vi "FLL Tournament Control.vi"() -> ()   [LabVIEW 2013]
uses:
  Team Data Array.ctl
  Team Data.ctl
  ScoreList.ctl
  Full Score Entry.ctl
  ScoreEntry.ctl
  Sound Info.ctl
  <vilib>/sound2/lvsound2.llb/Sound Data Format.ctl
  ImageInfoList.ctl
  TeamManager/TeamData_and_Schedule.ctl
  <vilib>/Utility/sysdir.llb/System Directory Type.ctl
  Logfile Entry.ctl
  Error File Queue Contents.ctl
  Score File Queue Contents.ctl
  <vilib>/sound2/lvsound2.llb/Sampling Mode.ctl
  Schedule Data.ctl
  <vilib>/Analysis/baseanly.llb/Mean (DBL).vi
  <vilib>/Utility/xml.llb/Write to XML File(string).vi
  Score Event Refnum.vi
  <vilib>/sound2/lvsound2.llb/Sound Output Set Volume (Single).vi
  <vilib>/sound2/lvsound2.llb/Sound Output Write (DBL).vi
  <vilib>/Platform/browser.llb/Open URL in Default Browser (string).vi
  <vilib>/Utility/xml.llb/Read From XML File(string).vi
  <vilib>/httpClient/LabVIEWHTTPClient.lvlib
  <vilib>/Analysis/NI_AALBase.lvlib
panel:
  in  "Local Entry Button":bool
  in  "Low Sponsor Image List":T1
  in  "Mid Sponsor Image List":T1
  in  "Top Sponsor Image List":T1
  in  "Profile Button":bool
  in  "Home Button":bool
  in  "System Monitor Button":bool
  in  "View Rankings Button":bool
  in  "Go to Timekeeper Button":bool
  in  "Launch Score Entry":bool
  in  "Settings Button":bool
  in  "Sound To Play":T2(ring)
  out "Sound Cluster":T3={"Start"={"total number of samples/ch"=31680, "sound format"={"sample rate (S/s)"=11025.0, "number of channels"=1, "bits per sample"=16}, "data"=[{"t0"=timestamp(0 s since 1904-01-01), "dt"=9.070294784580499e-05, "Y"=array[31680 elements]}], "Volume"=100.0}, "Stop"={"total number of samples/ch"=27648, "sound format"={"sample rate (S/s)"=11025.0, "number of channels"=1, "bits per sample"=16}, "data"=[{"t0"=timestamp(0 s since 1904-01-01), "dt"=9.070294784580499e-05, "Y"=array[27648 elements]}], "Volume"=100.0}, "Uh-Oh"={"total number of samples/ch"=29952, "sound format"={"sample rate (S/s)"=11025.0, "number of channels"=1, "bits per sample"=16}, "data"=[{"t0"=timestamp(0 s since 1904-01-01), "dt"=9.070294784580499e-05, "Y"=array[29952 elements]}], "Volume"=88.46153846153847}, "PreMatch"={"total number of samples/ch"=225792, "sound format"={"sample rate (S/s)"=44100.0, "number of channels"=2, "bits per sample"=16}, "data"=[{"t0"=timestamp(0 s since 1904-01-01), "dt"=2.2675736961451248e-05, "Y"=array[225792 elements]}, {"t0"=timestamp(0 s since 1904-01-01), "dt"=2.2675736961451248e-05, "Y"=array[225792 elements]}], "Volume"=75.38461538461539}, "Hurry-Up"={"total number of samples/ch"=0, "sound format"={"sample rate (S/s)"=0.0, "number of channels"=0, "bits per sample"=0}, "data"=[], "Volume"=0.0}}
  out "Table Names":string[](array[string])
  in  "Tab Control":T5(tab)=enum."Splash"
  out "Users String":string
  out "String 3":string="System Settings\n\nThis page is for Server System Settings.  \n\nTimer / Sounds - Press the button for \"Configure Sounds and Timer\" to set specific timer and sound properties.\n\nFile Paths - Don't change these unless you really know what you're doing.  If you change these, files will be saved or read from different locations than the \"default\" locations.  This may be good or bad, depending on the situation.  Beware.\n\nSecurity Entry Access Password - if you wish to put a password on the \"Web Entry\" score webpage, put the password here.  This value does not persist between software reboots.  The default value is \"321LEGO\".  When a user enters this password within the prompt when attempting to access a security-protected page, the user's \"system credentials\" are added to a Security Access List and attempts to access the software from that \"system\" no longer requires a password.  To clear out the access list and remove all users (for instance once you've set a new password to be used), press \"Clear Access List.\"  The local user ALWAYS has access."
  in  "Clear Access List Button":bool
  in  "Score Entry Access Password":string="321LEGO"
  in  "Team Data File Path":path=path "Z:/Code/LabVIEW/FLL 2.1/scorefile.xml"
  in  "Score Folder":path=path "Z:/Code/LabVIEW/FLL 2.1/Score Files"
  in  "Scoring Data File Path":path=path "Z:/Code/LabVIEW/FLL 2.1/scorefile.xml"
  in  "Timing Logfile Path":path=path "Z:/Code/LabVIEW/FLL 2.1/timing.log"
  in  "Error Folder":path=path "Z:/Code/LabVIEW/FLL 2.1/Error Files"
  in  "Error Logfile Path":path=path "Z:/Code/LabVIEW/FLL 2.1/error.log"
  in  "Scoring Logfile Path":path=path "Z:/Code/LabVIEW/FLL 2.1/scoring.log"
  in  "Schedule File Path":path=path "Z:/Code/LabVIEW/FLL 2.1/schedule.csv"
  in  "stop":bool
  in  "Configure Sounds Button":bool
  out "Timer Log":string[][](table)
  out "Scoring Log":string[][](table)
  out "Error Log":string[][](table)
  in  "PH 2":bool
  out "Score Queue Full":bool
  out "Error Queue Full":bool
  out "Write Scores to file indicator":bool
  out "Scores Exist":bool
  out "Teams Exist":bool
  out "Uh-Oh Sound Indicator":bool
  out "Stop Sound Indicator":bool
  out "Start Sound Indicator":bool
  out "Server Running":bool
  out "Web Pages Not Found":bool
  out "Log Queue Full":bool
  out "Network Interface Up":bool=TRUE
  out "PH":bool
  out "Port":string
  out "Current IP":string="192.168.0.3"
  in  "Delete Team":bool
  in  "Team Info":T6
  out "Number of Teams":i32
  in  "Score Entry":bool
  in  "Restore Session":bool
  in  "Input File Type":T8(radio)
  out "Number of Scores":i32
  in  "Replace Current Score Data\nFrom File":bool
  in  "Score File Path (Read)":path
  out "Score Data":T9 {"Score"."Score Mode Selector" items=["Automatic", "Manual"]}
  in  "Schedule To Show":enum16{"Practice", "Ranking"}(ring)=enum."Ranking"
  out "Schedule":i32(listbox)
  in  "Hurry-Up Sound Volume":dbl(slide)=88.46153846153847 scale=0.0..100.0
  in  "Hurry-Up Sound":path=path "Z:/Code/LabVIEW/FLL 2.1/sounds/FOGHORN.wav"
  out "mean":dbl format="%0.2f"
  out "min value":u32
  out "max value":u32
  in  "Boolean":bool
  in  "Secondary (s)":dbl
  in  "Primary (s)":dbl=150.0
  in  "Pre-Primary (s)":dbl
  in  "Test Pre-Match Sound":bool
  in  "Load Pre-Match Sound":bool
  in  "Pre-Match Coundown Sound Volume":dbl(slide)=88.46153846153847 scale=0.0..100.0
  in  "Pre-Match Countdown Sound":path=path "Z:/Code/LabVIEW/FLL 2.1/sounds/FOGHORN.wav"
  in  "Test Uh-Oh Sound":bool
  in  "Load Uh-Oh Sound":bool
  in  "Uh-Oh Sound Volume":dbl(slide)=88.46153846153847 scale=0.0..100.0
  in  "Uh-Oh Sound Path":path=path "Z:/Code/LabVIEW/FLL 2.1/sounds/FOGHORN.wav"
  in  "Test Stop Sound":bool
  in  "Load Stop Sound":bool
  in  "Stop Sound Volume":dbl(slide)=100.0 scale=0.0..100.0
  in  "Stop Sound Path":path=path "Z:/Code/LabVIEW/FLL 2.1/sounds/BUZZER.wav"
  in  "Test Start Sound":bool
  in  "Load Start Sound":bool
  in  "Start Sound Volume":dbl(slide)=100.0 scale=0.0..100.0
  in  "Start Sound Path":path=path "Z:/Code/LabVIEW/FLL 2.1/sounds/CHARGE.wav"
  in  "Master Volume":dbl(slide)=100.0 min=1.0 scale=0.0..100.0
  in  "Splash Page Main Tab Control":T12(tab)
  out "Welcome Text":string="Welcome to the FIRST LEGO League Tournament Software\nThis is RELEASE 2.0 of the software.  \nPlease test this software heavily before use to ensure familiarity.\n\nQUICK INTRODUCTION\n--------------------------\n\nThe FIRST LEGO League Tournament Software is a web-centric application.  It is designed to act as a SERVER which multiple CLIENTS can interact with simultaneously via exported web interfaces.  Therefore, this application only provides a bare minimum of services, but exposes its functionality via web pages that are served.\n\nPossible CLIENTS can be additional PCs connected to the same network, tablets or WiFi enabled devices connected via a wireless switch or router also on the same network as the computer running this application, or additional web-enabled devices running standard browsers with JavaScript enabled.  CLIENTS must use their web browser to connect to the IP Address, Port, and Service to access exported interfaces.  On the left of this text is a box marked, \"Web Interface Location\" which contains the full path that must be entered into a web browser to access a list of exported web interfaces to the FLL Tournament Software.  Pressing the \"LAUNCH\" button will launch a web browser and navigate to a main index of exported interfaces.\n\nNOTE:  It is vitally important to ensure that CLIENTS navigating to the Web Interface Location use the correct CASE, as the web path is CASE SENSITIVE.  \n\n\nSOFTWARE QUICK-START GUIDE\n-----------------------------------\n\nThe software requires very little in order to get started.  \n\n(0) Open and run this SERVER program\n(1) Follow on-screen prompts to start a new game or continue one in progress.\n(2) Enter Profile Info for your tournament - profile info auto-saves.\n(3) Open display and connect to server\n(4) Launch a web browser session and use the software!\n\nTournaments have two choices for getting team and schedule information into the software; (1) using the traditional method of using a schedule file generated by Bryan Lee's Excel tool, and (2) creating and editing a team list manually.  Tournaments who choose to create/edit a team list manually will generally do so because they did not use Bryan Lee's software to generate a schedule for them, and typically already have a schedule that the tournament will use.  This software DOES NOT generate schedules, but if you've used Bryan Lee's tool to generate one you can import it.\n\n\nTOURNAMENT TEAM LISTS AND SCHEDULES\n-------------------------------------------------\n\nThe minimum amount of information required to run a tournament is a list of teams to use for score input and display.  The software now provides a utility for creating this slimmed-down information, and it can be found on the HOME page when creating a new tournament and accessed via the \"Create / Edit Team List\" button.  However, tournaments also have the option of using Bryan Lee's Excel Tournament Schedule Generator, and this software is capable of importing the CSV export created by that software.  Once teams and schedules are imported into the software from the CSV export, teams may also be edited using the \"Edit Team List\" button - however, any changes made are NOT reflected back to the CSV file; any changes are local-only.\n\nThis Tournament Software provides facilities for showing the tournament schedule details to emcees/announcers and competition staff if that functionality is so desired.  Since this software DOES NOT generate schedules, this functionality is not available to tournaments who use the simple team list generation method provided by this software.  \n\n\nEXPLANATION OF SOFTWARE NAVIGATION BUTTONS\n----------------------------------------------------------\n\nThe buttons along the bottom of the application are meant to be used to quickly navigate to various areas of the tournament software.  You can always get back to this screen by clicking on the \"HOME\" button with the \"house\" graphic.  A description of each button is as follows:\n\nHOME - The \"home\" button signified by the \"house\" icon brings you back to this guide.  Navigating back to this guide in no way compromises or harms the operation of the scoring software.\n\nWEB ENTRY - The FLL Tournament Software was designed to be web-centric; as such, there is no built-in  score entry mechanism within this software.  By pressing the \"Web Score\" button, the default browser for this computer will be launched and automatically navigated to a score entry web page.  This web page is the same one that is \"served\" to external clients.  Multiple score entry stations may operate simultaneously by using this web input method.\n\nLOCAL ENTRY - The FLL Tournament Software has the ability to allow a SINGLE station (the local server station) to manually edit scores.  The theory behind this is that it's quick and easy to enter in a score, so a single person should be able to handle it with ease.  Plus it didn't make sense to turn this into a web page.\n\nTIMER - The timekeeper mechanism is the local timekeeper portal, and also manages the current match number and the tournament phase.  This software was designed for the web, so there is also a web portal for accessing and controlling the timer via external clients.  Only the local timekeeper client within this application has the ability to modify the current match number.\n\nRANK - The rankings page allows tournament staff to view the current team rankings.  Tournaments may choose to require \"multiple validation\" and may set the number of duplicate validations for a given match before posting the score.  This is useful for tournaments concerned about data entry, and allows the score to be entered and validated by multiple individuals before being shown.\n\nSTATUS - The FLL Tournament Software is a complex piece of software, and the STATUS page provides a quick summary of the state of the software.  Let's leave it at that for now.\n\nSETTINGS - The settings page provides all of the necessary path, configuration information, and relevant settings for the Tournament Software.  This still needs to be heavily modified.\n\nPROFILE - The profile page is where you customize the software for your tournament, to give it a name, to import logos, and so on.  If you play 4 rounds at your tournament, this is the place to specify 3 rounds or 4 rounds.  Understand that the score page will not likely update immediately when changes are made, but when the page is refreshed (each time the scores cycle through, generally, or the logos cycle for the largest logo set)."
  out "String 2":string="Timekeeper Mode\n\nUnfortunately changing the phase does nothing right now, so it's disabled.  This software is currently only a single-mode program; if you submit \"practice\" scores, you must close the software and restart a new game in order to submit \"ranking\" scores.\n\nYou can use the Start / Stop buttons to start and stop the timer, or use the web interface to do the same thing.  You can also adjust the current match by using the Previous / Next buttons to Decrement / Increment the match number, respectively."
  out "Time Remaining":string
  in  "Timer Stop":bool
  in  "Timer Start":bool
  in  "Next Match":bool
  in  "Previous Match":bool
  out "Current Match":u16=1
  in  "Current Phase":enum16{"Practice", "Ranking"}(ring)=enum."Ranking"
  out "Team Rankings":string[][](table)
  in  "Needed Validations":u16=1 min=1
  in  "Write Score Data To Human-Readable CSV File":bool
  in  "SUBMIT Manual Score":bool
  in  "ROUND":u16(ring) items=["1", "2", "3", "4"]
  in  "Select a Team for Manual Score Entry":u16(ring) items=["1, Green Man Group", "15, EOT (prounced E-OH-TE)", "23, ROBOWhizards", "32, Fire Breathing Rubber", "58, Gear Geeks", "87, W.A.F.F.L.E.S.", "105, Crusaders", "127, Whitney Killer Watts", "131, The Brainy Bunch", "165, RoboRaiders", "171, Fossil Fuel Fighters", "223, FellowshipOfTheBricks", "299, Bearbotics", "334, Power Peeps", "426, Gothic Lawn Gnomes", "482, Lego Guards", "543, SCS Penguins", "548, Damsels in Charge", "606, Longhorn Robotics", "654, Central SpaceLab ONE", "857, NRG Bots", "995, Roboteers", "1133, Power Pirates", "1409, St. Clare's School", "1413, Terramatix", "1490, FOLSOM GATOROBYTES", "1523, Mindstorm Maniacs", "1579, SWAT (Superior Workin)", "1582, Energizer Eagles", "1592, Electrolights", "1832, Techno Warriors", "1976, The Inventioneers", "2093, Transformers", "2254, Landroids", "2430, The Blue Dragons", "2560, Pixelation", "2721, Nuclear Knights", "2744, The Oddly Charged Par", "2765, NeXT GEN", "2822, Techno Beasts", "2866, Cobalt Blue", "2922, Alternative Robotics Team", "2927, Storm Cats", "3162, Laser Blazers", "3267, Legooners", "3430, Robo - Monkey - Kilts", "3456, Lightning Rod", "3457, Rainstorm Robotics", "3492, Logos Legos", "3753, CYBORGS", "4049, Solar Dragons", "4198, Ridgewood Robo Raider", "5321, Lights Out", "5746, Super Battle Droids", "5947, Highlanders", "7105, Team LEET", "8000, Junior Kids", "8005, Alleskönner?!", "8010, Herta-Mechanics", "8015, Montfort-Robot", "8035, COMPLUBOT", "8040, Terakki", "8045, TSM Roboteam UK", "8050, SAP NXTreme", "8055, Techno Future Egypt", "8060, The Legoroos", "8065, EAST ASIAN STAR ", "8070, SAP SpIDERs", "8075, Formula Green", "8080, Eleven", "8085, CREATIVE ENGINEERS", "8090, Sizars", "8095, External Fusion", "8100, Danger Mind", "8110, BLACK OCEAN CURRENT", "8120, Nucleólicos", "8125, POWERGENESIS", "8130, MDLB108", "8131, Campeones FNH", "8135, ROBOOG Challenge team", "8140, Save Earth", "9000, FIRST Team - Fill in"]
  out "String":string="Manual Score Entry\n\nThis is intended to ONLY be used to enter manual scores into the system.  Overriding a calculated score (one entered via the Web Entry) will destroy all record of what was entered to calculate the score.  This mode does not attempt to validate the score.  \n\nTo submit a manual score, select the team to receive the score.  The team field must be changed in order to activate the \"Submit\" button - this might require selecting a different team and coming back (on the first team entered or when entering scores for the same team in succession) - this is a protection feature to keep you from accidentally setting a score on a team by accident.  Then select the ROUND that this score will apply to; the ROUND will be automatically selected to the next empty ROUND for the selected team, but any match may be selected.  Once the round is selected, enter the MATCH SCORE for the team, and then press SUBMIT."
  in  "Manual Score":dbl
  in  "Startup Navigation Tab Control":enum32{"Start", "New", "Done"}(tab)
  out "Dumb Text Prompt 1":string="Welcome!  We can start a New Game or we can continue a Game in Progress.  Which would you like to do?\n\nPlease click one of the below options..."
  in  "Start New Game Button":bool
  in  "Continue Game Button":bool
  in  "New Game Back Button":bool
  in  "Load Schedule Button":bool
  in  "Create/Edit Team List":bool
  out "Dumb Text Prompt 2":string="Shall we load a Schedule .csv Export File from Bryan Lee's Tournament Scheduler, or create our own team list?"
  out "Web Interface Location":string
  in  "Launch Web Server Button":bool
  in  "Edit Team Information Button":bool
  in  "Rounds to Show":u16(ring) items=["Three", "Four"]
  out "Preview":picture
  in  "Main Logo Image (129x462)":path
  in  "Display Screen Title":string="Central Texas FIRST LEGO League"
  in  "Config Low Sponsors Button":bool
  in  "Config Mid Sponsors Button":bool
  in  "Config Top Sponsors Button":bool
  # "Not implemented, and doesn't have to be! Wheee!"
  # "SYSTEM RECOVERY"
  # "1. Set \"Team Data File Path,\" \"Scoring Data File Path,\"\nand \"Schedule File Path\" to appropriate files.\n2. Press \"Go.\""
  # "5"
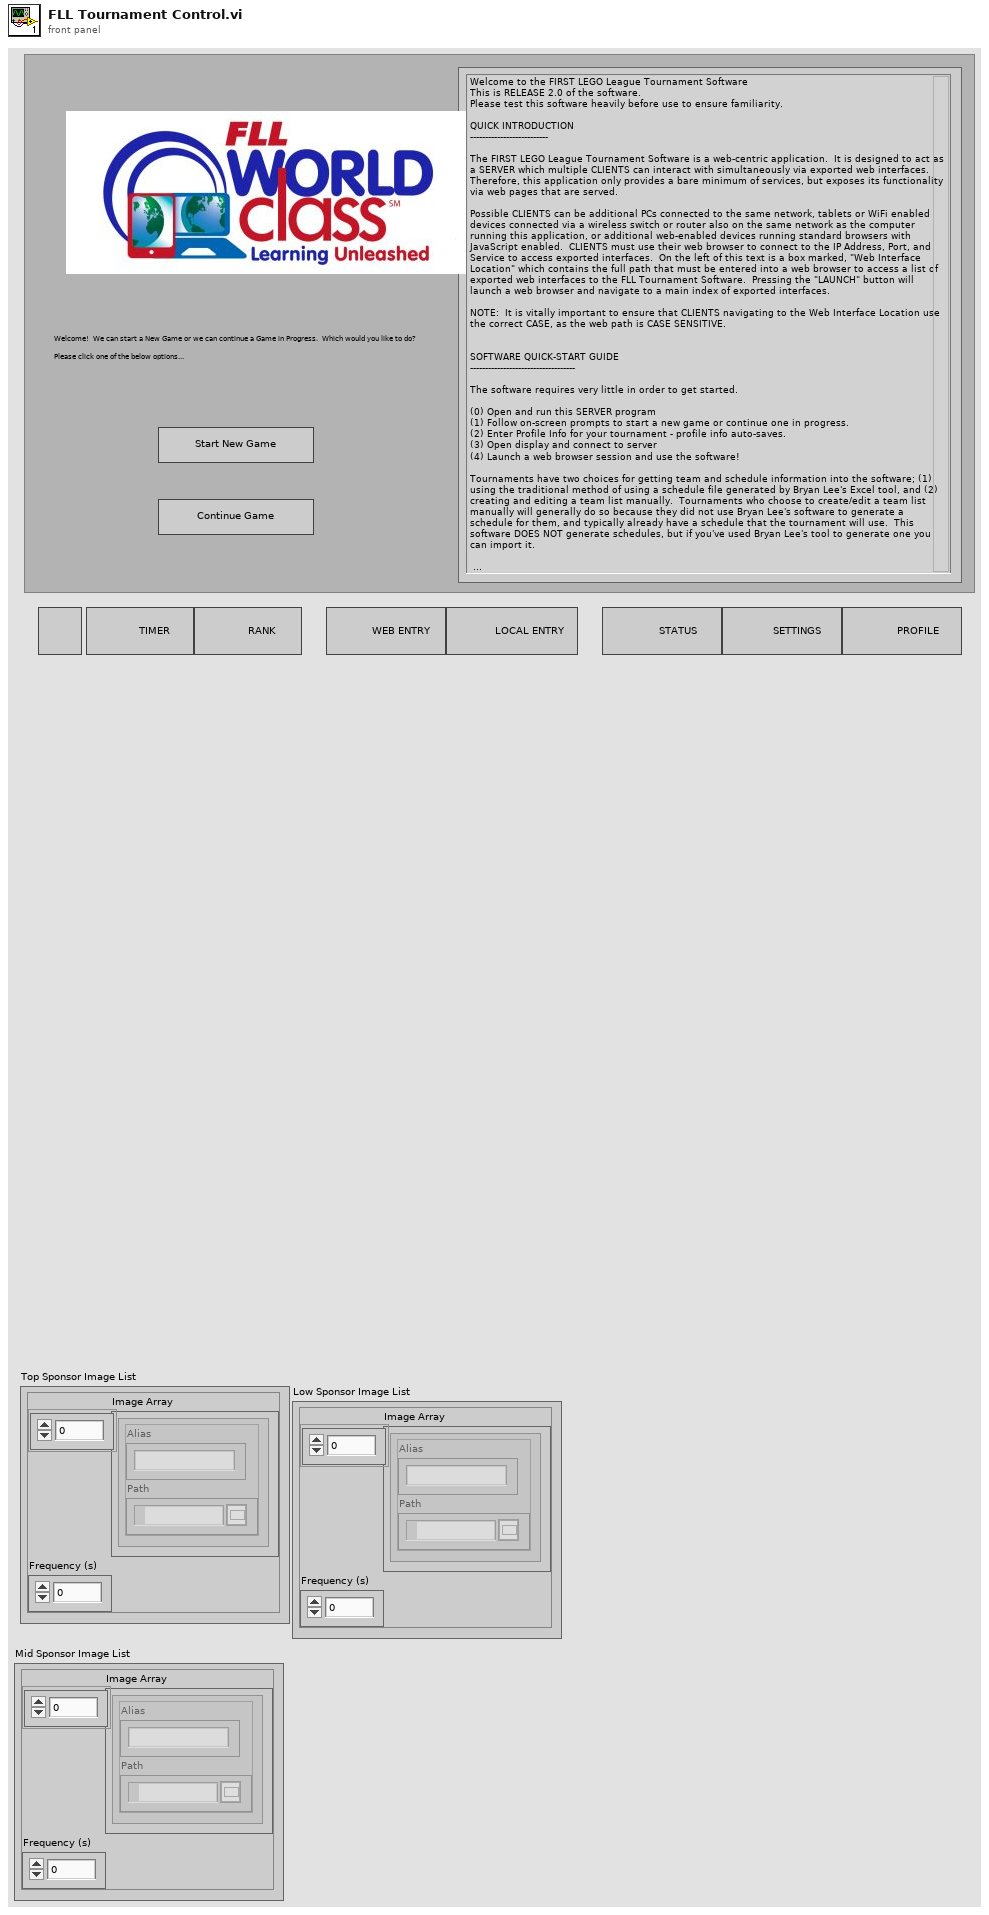
[diagram p1: front panel]
types:
  T1 = typedef "ImageInfoList.ctl" = cluster{"Image Array":cluster{"Alias":string, "Path":path}[], "Frequency (s)":dbl}
  T2 = enum16{"None", "Start", "Stop", "Uh-Oh", "Prematch", "Hurry-Up"}
  T3 = typedef "Sound Info.ctl" = cluster{"Start":cluster{"total number of samples/ch":u32, "sound format":T4, "data":waveform(dbl)[], "Volume":dbl}, "Stop":cluster{"total number of samples/ch":u32, "sound format":T4, "data":waveform(dbl)[], "Volume":dbl}, "Uh-Oh":cluster{"total number of samples/ch":u32, "sound format":T4, "data":waveform(dbl)[], "Volume":dbl}, "PreMatch":cluster{"total number of samples/ch":u32, "sound format":T4, "data":waveform(dbl)[], "Volume":dbl}, "Hurry-Up":cluster{"total number of samples/ch":u32, "sound format":T4, "data":waveform(dbl)[], "Volume":dbl}}
  T4 = typedef "Sound Data Format.ctl" = cluster{"sample rate (S/s)":dbl, "number of channels":i32, "bits per sample":i32}
  T5 = enum32{"System Control", "System Monitor", "Timer Control", "Team Control", "Local Score Entry", "Score Control", "Schedule", "Rankings", "Experimental", "Splash", "Profiles"}
  T6 = typedef "Team Data Array.ctl" = T7[]
  T7 = typedef "Team Data.ctl" = cluster{"Both":string, "Name":string, "GUID":u16, "Number":u16}
  T8 = enum32{"Human Readable XML", "LabVIEW Flat XML", "Build From Score Files"}
  T9 = typedef "ScoreList.ctl" = cluster{"ValidationCount":u16, "Score":T10}[]
  T10 = typedef "Full Score Entry.ctl" = cluster{"GUID":u16, "Score Mode Selector":u16, "Round Number":u16, "Full Score Entry":T11}
  T11 = typedef "ScoreEntry.ctl" = cluster{"Elements":cluster{"Name":string, "Value":string}[], "Score":dbl}
  T12 = enum32{"Main Splash Instructions", "Timekeeper", "Rankings", "Manual Score Entry"}
  T13 = enum16{"Get Teams", "Add Team", "Modify Team", "Clear All Teams", "Force Add Team", "Delete Team"}
  T14 = enum16{"Get Timer State", "Start Timer", "Stop Timer"}
  T15 = enum16{"Get", "Increment", "Decrement", "Set Match", "Set Phase"}
  T16 = enum16{"Stopped", "Primary", "Secondary", "Pre-Primary"}
  T17 = enum32{"Main Splash Instructions", "Timekeeper", "Rankings"}
  T18 = enum32{"System Control", "System Monitor", "Timer Control", "Team Control", "Local Score Entry", "Score Control", "Schedule", "Rankings", "Experimental", "Splash"}
  T19 = typedef "System Directory Type.ctl" = i32
  T20 = cluster{"Master Volume":dbl, "Pre-Primary (s)":dbl, "Primary (s)":dbl, "Secondary (s)":dbl, "Start Sound Path":path, "Stop Sound Path":path, "Uh-Oh Sound Path":path, "Pre-Match Countdown Sound":path, "Hurry Up Sound":path, "Start Sound Volume":dbl, "Stop Sound Volume":dbl, "Uh-Oh Sound Volume":dbl, "Pre-Match Coundown Sound Volume":dbl, "Hurry Up Sound Volume":dbl}
  T21 = enum8{"Enabled", "Disabled", "Disabled and Grayed Out"}
  T22 = typedef "imagedata.ctl" = cluster{"image type":i32, "image depth":i32, "image":u8[], "mask":u8[], "colors":u32[], "Rectangle":cluster{"left":i16, "top":i16, "right":i16, "bottom":i16}}
  T23 = typedef "Schedule Data.ctl" = cluster{"Practice Matches":string[][], "Ranking Matches":string[][], "Table Names":string[], "Ranking Match Times":string[][], "Practice Match Times":string[][]}
  T24 = enum16{"Get Teams", "Add Team", "Modify Team", "Clear All Teams"}
  T25 = enum32{"System Control", "System Monitor", "Timer Control", "Team Control", "Local Score Entry", "Score Control", "Schedule", "Rankings", "Experimental"}
  T26 = enum16{"open", "replace", "create", "open or create", "replace or create", "replace or create with confirmation"}
  T27 = cluster{"total number of samples/ch":u32, "sound format":T4, "data":waveform(dbl)[], "Volume":dbl}
  T28 = cluster{"GUID":u16, "Team Number":u16, "Team Name":string, "Highest Score":dbl, "Scores":cluster{"Score":dbl, "Round":u16}[]}[]
  T29 = enum16{"Left Button", "Center Button", "Right Button", "Window Close"}
  T30 = typedef "LabVIEWHTTPClient.lvlib/ClientHandle.ctl" = refnum<k1>
  T31 = typedef "Sampling Mode.ctl" = i32
  T32 = typedef "Sound Output Task ID.ctl" = u32
  T33 = cluster{"Primary":dbl, "Secondary":dbl, "Pre-Primary":dbl}
  T34 = enum16{"Logo Path", "Logo", "Title", "Rounds", "LastSound"}
  T35 = enum16{"None", "Start", "Stop", "Uh-Oh", "Prematch"}
  T36 = typedef "Score File Queue Contents.ctl" = cluster{"Scoring Data":cluster{"Name":string, "Value":string}[], "Round":u16, "GUID":u16, "GUSID":string, "Time Stamp":timestamp, "Submitter":string}
  T37 = typedef "Error File Queue Contents.ctl" = cluster{"Filename":string, "File Contents":string, "Time Stamp":timestamp, "Origin":string}
  T38 = typedef "Logfile Entry.ctl" = cluster{"Time Stamp":timestamp, "Origin":string, "Message":string, "Log":enum16{"Error Log", "Timer Log", "Scoring Log"}}
  T39 = enum16{"Get Teams", "Add Team", "Modify Team", "Clear All Teams", "Force Add Team", "Delete Team", "Add Team With GUID"}
  T40 = typedef "TeamData_and_Schedule.ctl" = cluster{"Team Info":cluster{"Number":u16, "Both":string, "Name":string, "GUID":u16}[], "Match Array (indices)":i32[][]}
  T41 = cluster{"Number":u16, "Both":string, "Name":string, "GUID":u16}[]
  T42 = cluster{"Team Info[0]":cluster{"Number":u16, "Both":string, "Name":string, "GUID":u16}}
  T43 = cluster{"Number":u16, "Both":string, "Name":string, "GUID":u16}
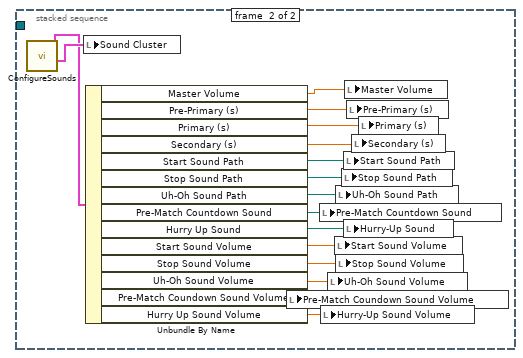
[diagram p2: hidden frame]
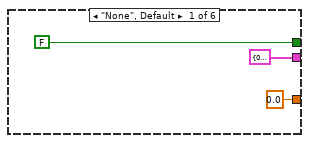
[diagram p4: hidden frame]
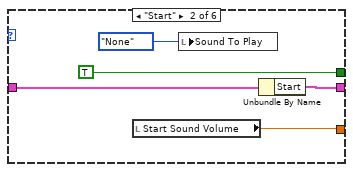
[diagram p5: hidden frame]
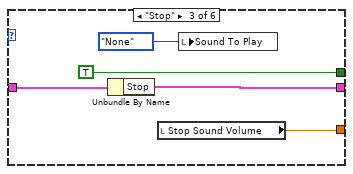
[diagram p6: hidden frame]
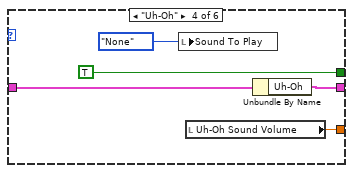
[diagram p7: hidden frame]
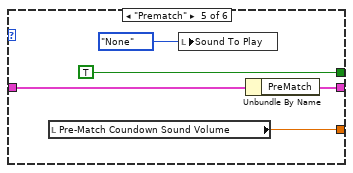
[diagram p8: hidden frame]
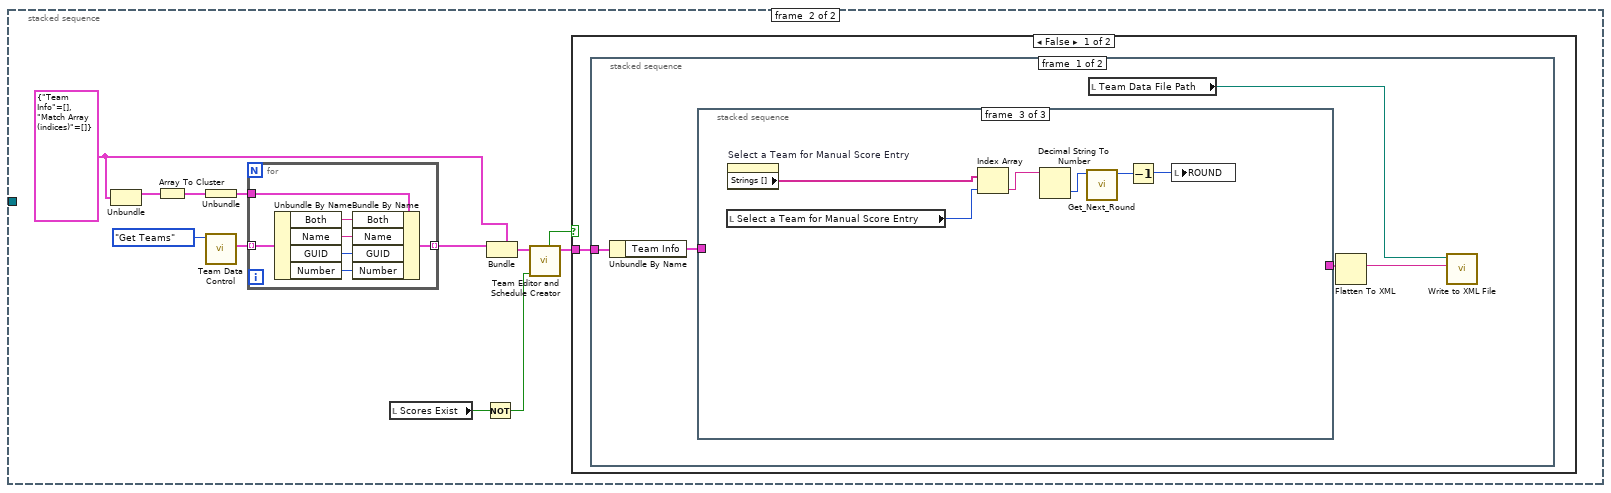
[diagram p9: hidden frame]
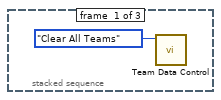
[diagram p10: hidden frame]
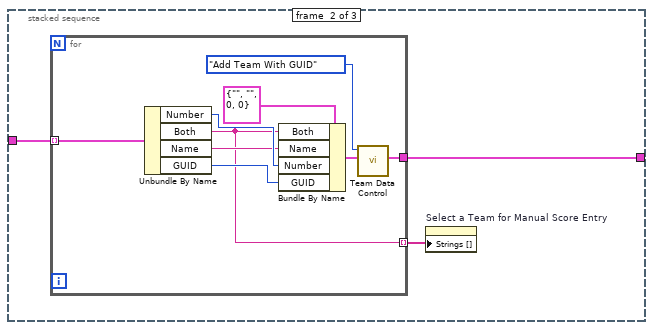
[diagram p11: hidden frame]
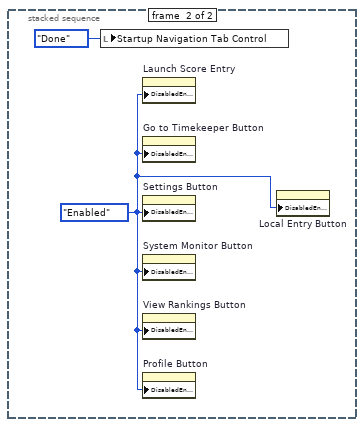
[diagram p12: hidden frame]
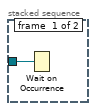
[diagram p14: hidden frame]
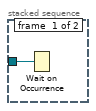
[diagram p15: hidden frame]
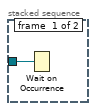
[diagram p16: hidden frame]
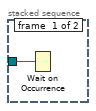
[diagram p17: hidden frame]
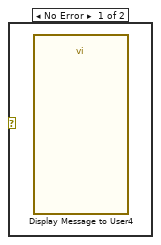
[diagram p18: hidden frame]
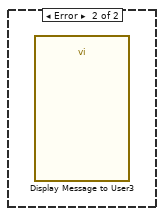
[diagram p19: hidden frame]
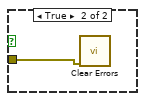
[diagram p20: hidden frame]
diagram:
  n1 = stacked-sequence "Init" {
    tunnel: [_ _ _ _ _ _ _ w128] -> w6
    tunnel: [w15 _ _ _ _ _ _ _] -> w13
    frame #0 {
      w16 = TRUE  # Is Changed
      # "Create score change event"
      n2 = Create User Event(user event datatype=w16) -> (user event=w15:refnum<user-event>)  [unwired: 1 in, 1 out]
      n3 = global write "Score Event Refnum.vi" "user event out"(w15) -> ()
    }
    frame #1 {
      n4 = disable-structure shown="RUN_TIME_ENGINE==False" {
        disable-tunnel: ["8008" ("string") "8001" ("string")] -> w17
        frame condition #0 {
        }
        frame condition #1 (active) {
        }
      }
      n5 = local write "Port"(w17) -> ()
    }
    frame #2 {
      w43 = T19 7 items=["User Home"=0, "User Desktop"=1, "User Documents"=2, "User Application Data"=3, "User Preferences"=4, "User Temporary"=5, "Public Documents"=6, "Public Application Data"=7, "Public Preferences"=8, "Public Cache"=13, "System Core Libraries"=9, "System Installed Libraries"=10, "Application Files"=11, "Boot Volume Root"=12] ("system directory type")
      n6 = call <vilib>:"Get System Directory.vi"("create directory if not found? (F)"=TRUE, "system directory type"=w43) -> ("system directory"=w41:path)  [unwired: 9 in]
      n7 = Build Path(base path=w41, name or relative path="FLL") -> (appended path=w39:path)
      n8 = call "Check and Create Folder.vi"("appended path"=w39) -> ("dup path"=w33:path)  [unwired: 10 in]
      n9 = Build Path(base path=w33, name or relative path="profile.xml") -> (appended path=w32:path)
      n10 = call <vilib>:"Check if File or Folder Exists.vi"("path"=w32) -> ("file or folder exists?"=w36:bool, "dup path"=w35:path)  [unwired: 8 in, 1 out]
      n11 = case shown="True" w36 {
        tunnel: [w65 w91] -> w51
        tunnel: [w64 w91] -> w50
        tunnel: [w66 w91] -> w49
        tunnel: [w88 w91] -> w48
        tunnel: [w86 w91] -> w30
        tunnel: [w84 w91] -> w47
        tunnel: [w82 w91] -> w46
        tunnel: [w80 w91] -> w45
        tunnel: [w75 w91] -> w44
        tunnel: w33 -> [w72 _]
        tunnel: [w69 w91] -> w38
        tunnel: [w68 w91] -> w37
        tunnel: w35 -> [_ _]
        tunnel: [w63 w91] -> w31
        tunnel: [w62 w91] -> w29
        tunnel: [w60 w90] -> w28
        tunnel: [w59 w90] -> w27
        tunnel: [w58 w90] -> w26
        tunnel: [w57 w90] -> w25
        tunnel: [w56 w90] -> w24
        tunnel: [w55 w90] -> w23
        tunnel: [w54 w90] -> w22
        tunnel: [w53 w90] -> w21
        tunnel: [w52 w90] -> w20
        frame False {
          n12 = call "GetConfiguredSounds.vi"() -> ("Sound Cluster"=w61:T3, "Settings Cluster"=w67:T20)  [unwired: 10 in]
          n13 = Unbundle By Name(w67) -> ("Master Volume"=w60:dbl, "Pre-Primary (s)"=w59:dbl, "Primary (s)"=w58:dbl, "Secondary (s)"=w57:dbl, "Start Sound Path"=w65:path, "Stop Sound Path"=w64:path, "Uh-Oh Sound Path"=w66:path, "Pre-Match Countdown Sound"=w63:path, "Hurry Up Sound"=w62:path, "Start Sound Volume"=w56:dbl, "Stop Sound Volume"=w55:dbl, "Uh-Oh Sound Volume"=w54:dbl, "Pre-Match Coundown Sound Volume"=w53:dbl, "Hurry Up Sound Volume"=w52:dbl)
          n14 = local write "Sound Cluster"(w61) -> ()
          n15 = Build Path(base path=w72, name or relative path="schedule.csv") -> (appended path=w86:path)
          n16 = Build Path(base path=w72, name or relative path="Score Files") -> (appended path=w71:path)
          n17 = Build Path(base path=w72, name or relative path="Error Files") -> (appended path=w70:path)
          n18 = Build Path(base path=w72, name or relative path="Data") -> (appended path=w74:path)
          n19 = call "Check and Create Folder.vi"("appended path"=w71) -> ("dup path"=w68:path)  [unwired: 10 in]
          n20 = call "Check and Create Folder.vi"("appended path"=w70) -> ("dup path"=w69:path)  [unwired: 10 in]
          n21 = call "Check and Create Folder.vi"("appended path"=w74) -> ("dup path"=w73:path)  [unwired: 10 in]
          n22 = Build Path(base path=w73, name or relative path="scorefile.xml") -> (appended path=w88:path)
          n23 = Build Path(base path=w73, name or relative path="teamfile.xml") -> (appended path=w75:path)
          n24 = Build Path(base path=w73, name or relative path="scoring.log") -> (appended path=w82:path)
          n25 = Build Path(base path=w73, name or relative path="error.log") -> (appended path=w84:path)
          n26 = Build Path(base path=w73, name or relative path="timing.log") -> (appended path=w80:path)
        }
        frame True {
          w90 = 0.0
          w91 = path ""
        }
      }
      n27 = local write "Secondary (s)"(w25) -> ()
      n28 = local write "Master Volume"(w28) -> ()
      n29 = local write "Uh-Oh Sound Volume"(w22) -> ()
      n30 = local write "Pre-Match Coundown Sound Volume"(w21) -> ()
      n31 = local write "Pre-Primary (s)"(w27) -> ()
      n32 = local write "Start Sound Volume"(w24) -> ()
      n33 = local write "Stop Sound Volume"(w23) -> ()
      n34 = local write "Primary (s)"(w26) -> ()
      n35 = local write "Hurry-Up Sound Volume"(w20) -> ()
      n36 = local write "Pre-Match Countdown Sound"(w31) -> ()
      n37 = local write "Hurry-Up Sound"(w29) -> ()
      n38 = local write "Schedule File Path"(w30) -> ()
      n39 = local write "Team Data File Path"(w44) -> ()
      n40 = local write "Scoring Data File Path"(w48) -> ()
      n41 = local write "Scoring Logfile Path"(w46) -> ()
      n42 = local write "Error Logfile Path"(w47) -> ()
      n43 = local write "Timing Logfile Path"(w45) -> ()
      n44 = local write "Score Folder"(w37) -> ()
      n45 = local write "Error Folder"(w38) -> ()
      n46 = local write "Uh-Oh Sound Path"(w49) -> ()
      n47 = local write "Start Sound Path"(w51) -> ()
      n48 = local write "Stop Sound Path"(w50) -> ()
    }
    frame #3 {
      w97 = u16 2 items=["Get All", "Set", "Reset All", "Force Set"] ("Get/Set Mode Selector")
      # "Initialize func globs"
      n49 = call "ScoreControl.vi"("Get/Set Mode Selector"=w97) -> ()  [unwired: 13 in, 2 out]
      n50 = stacked-sequence {
        frame #0 {
          n51 = call "Timer Running Control.vi"("Enum"=T14."Stop Timer") -> ()  [unwired: 10 in, 1 out]
        }
        frame #1 {
          n52 = call "Current Match Control.vi"("New Phase"=enum16{"Practice", "Ranking"}."Ranking", "Mode"=T15."Set Phase") -> ("Current Phase"=w102:enum16{"Practice", "Ranking"})  [unwired: 8 in, 1 out]
          n53 = local write "Current Phase"(w102) -> ()
        }
        frame #2 {
          n54 = call "State Control.vi"("State"=T16."Pre-Primary", "Action"=enum16{"Get", "Set"}."Set") -> ()  [unwired: 9 in, 1 out]
        }
        frame #3 {
          n55 = local read "Pre-Primary (s)"() -> (w106:dbl)
          n56 = call "Time Remaining Control.vi"("Numeric"=w106, "Mode"=enum16{"Get", "Set"}."Set") -> ()  [unwired: 9 in, 1 out]
        }
        frame #4 {
          n57 = call "Current Match Control.vi"("New Match"=u16 1 ("Numeric"), "Mode"=T15."Set Match") -> ("Current Match"=w108:u16)  [unwired: 8 in, 1 out]
          n58 = local write "Current Match"(w108) -> ()
        }
      }
      n59 = call "Team Data Control.vi"("Mode"=T13."Clear All Teams") -> ()  [unwired: 10 in, 1 out]
      n60 = local write "Sound To Play"(enum16{"None", "Start", "Stop", "Uh-Oh"}."None" ("Sound To Play")) -> ()
      n61 = call "styles.css.vi"("Boolean"=FALSE, "Web"=FALSE, "Mode"=enum16{"G", "S", "T"}."S") -> ()  [unwired: 8 in, 1 out]
      n62 = call "GUID Allocator.vi"("Reinit GUID (Danger!)"=TRUE) -> ()  [unwired: 10 in, 1 out]
    }
    frame #4 {
      # "Initialize indicators"
      n63 = local write "Scoring Log"(string[][] [] ("Scoring Log")) -> ()
      n64 = local write "Error Log"(string[][] [] ("Error Log")) -> ()
      n65 = local write "Timer Log"(string[][] [] ("Event Log")) -> ()
      n66 = local write "PH"(FALSE ("PH")) -> ()
    }
    frame #5 {
      n67 = property on="Schedule" class="MCListbox (strict)"("ItemNames"=string[][] []) -> ()  [unwired: 2 in, 2 out]
      n68 = local write "Startup Navigation Tab Control"(enum32{"Start", "New", "Done"}."Start" ("Startup Navigation Tab Control")) -> ()
      n69 = local write "Tab Control"(T18."Splash" ("Tab Control")) -> ()
      n70 = local write "Splash Page Main Tab Control"(T17."Main Splash Instructions" ("Splash Page Main Tab Control")) -> ()
    }
    frame #6 {
      w119 = FALSE
      w118 = T21."Disabled and Grayed Out" ("Disabled")
      n71 = property on="Profile Button" class="Bool (strict)"("DisabledEnum"=w118) -> ()  [unwired: 2 in, 2 out]
      n72 = property on="Settings Button" class="Bool (strict)"("DisabledEnum"=w118) -> ()  [unwired: 2 in, 2 out]
      n73 = property on="Local Entry Button" class="Bool (strict)"("DisabledEnum"=w118) -> ()  [unwired: 2 in, 2 out]
      n74 = property on="View Rankings Button" class="Bool (strict)"("DisabledEnum"=w118) -> ()  [unwired: 2 in, 2 out]
      n75 = property on="Launch Score Entry" class="Bool (strict)"("DisabledEnum"=w118) -> ()  [unwired: 2 in, 2 out]
      n76 = property on="Go to Timekeeper Button" class="Bool (strict)"("DisabledEnum"=w118) -> ()  [unwired: 2 in, 2 out]
      n77 = property on="SUBMIT Manual Score" class="Bool (strict)"("DisabledEnum"=w118) -> ()  [unwired: 2 in, 2 out]
      n78 = property on="System Monitor Button" class="Bool (strict)"("DisabledEnum"=w118) -> ()  [unwired: 2 in, 2 out]
      n79 = local write "Config Low Sponsors Button"(w119) -> ()
      n80 = local write "Config Top Sponsors Button"(w119) -> ()
      n81 = local write "Config Mid Sponsors Button"(w119) -> ()
      n82 = call "Current Match Control.vi"("New Match"=u16 1 ("Numeric"), "Mode"=T15."Set Match") -> ("Current Match"=w121:u16)  [unwired: 8 in, 1 out]
      n83 = local write "Current Match"(w121) -> ()
    }
    frame #7 {
      w128 = FALSE ("stop")
      n84 = call "LoadImageListFromXML.vi"("filename"="topsponsors.xml") -> ("Top Sponsor Image List"=w127:T1)  [unwired: 10 in]
      n85 = call "LoadImageListFromXML.vi"("filename"="midsponsors.xml") -> ("Top Sponsor Image List"=w126:T1)  [unwired: 10 in]
      n86 = call "LoadImageListFromXML.vi"("filename"="lowsponsors.xml") -> ("Top Sponsor Image List"=w125:T1)  [unwired: 10 in]
      n87 = call "GetSetProfileInfo.vi"("Get/Set State"=enum16{"Get", "Set", "Load"}."Load") -> ("Logo Path Out"=w129:path, "Title"=w132:string, "image data out"=w130:T22)  [unwired: 6 in, 2 out]
      n88 = control-ref of="Preview"() -> (w131:refnum<vi>)
      n89 = local write "Top Sponsor Image List"(w127) -> ()
      n90 = local write "Mid Sponsor Image List"(w126) -> ()
      n91 = local write "Low Sponsor Image List"(w125) -> ()
      n92 = local write "Main Logo Image (129x462)"(w129) -> ()
      n93 = local write "Display Screen Title"(w132) -> ()
      n94 = call "Score Display - Display Image (LV).vi"("image data"=w130, "Picture Reference"=w131) -> ()  [unwired: 2 in]
      n95 = local read "Score Entry Access Password"() -> (w123:string)
      n96 = call "password.vi"("Action"=enum16{"Compare", "Set"}."Set", "password"=w123) -> ()  [unwired: 9 in, 1 out]
      n97 = local write "stop"(w128) -> ()
    }
  }
  n98 = Generate Occurrence() -> (w5:refnum<k4>)
  n99 = Generate Occurrence() -> (w4:refnum<k4>)
  n100 = Generate Occurrence() -> (w3:refnum<k4>)
  n101 = Generate Occurrence() -> (w2:refnum<k4>)
  n102 = Generate Occurrence() -> (w1:refnum<k4>)
  n103 = register-events(w13) -> (reference out=w14:refnum<event-registration>)  [unwired: 2 in, 1 out]
  n104 = while {
    tunnel: w5 -> [w137]
    stop <- w138 stop-if-true
    n105 = stacked-sequence {
      tunnel: w137 -> [w139 _]
      frame #0 {
        n106 = Wait on Occurrence(2:w139) -> ()  [unwired: 2 in, 1 out]
      }
      frame #1 {
        n107 = local read "Top Sponsor Image List"() -> (w143:T1)
        n108 = call "ImageListManager.vi"("filename"="topsponsors.xml", "Header Title String"="Top Sponsor Image List", "Image Information In"=w143) -> ("Image Information Out"=w142:T1)  [unwired: 8 in]
        n109 = local write "Top Sponsor Image List"(w142) -> ()
      }
    }
    n110 = local read "stop"() -> (w138:bool)
  }
  n111 = while {
    tunnel: w4 -> [w144]
    stop <- w145 stop-if-true
    n112 = stacked-sequence {
      tunnel: w144 -> [w146 _]
      frame #0 {
        n113 = Wait on Occurrence(2:w146) -> ()  [unwired: 2 in, 1 out]
      }
      frame #1 {
        n114 = local read "Mid Sponsor Image List"() -> (w150:T1)
        n115 = call "ImageListManager.vi"("filename"="midsponsors.xml", "Header Title String"="Mid Sponsor Image List", "Image Information In"=w150) -> ("Image Information Out"=w149:T1)  [unwired: 8 in]
        n116 = local write "Mid Sponsor Image List"(w149) -> ()
      }
    }
    n117 = local read "stop"() -> (w145:bool)
  }
  n118 = while {
    tunnel: w3 -> [w151]
    stop <- w152 stop-if-true
    n119 = stacked-sequence {
      tunnel: w151 -> [w153 _]
      frame #0 {
        n120 = Wait on Occurrence(2:w153) -> ()  [unwired: 2 in, 1 out]
      }
      frame #1 {
        n121 = local read "Low Sponsor Image List"() -> (w157:T1)
        n122 = call "ImageListManager.vi"("filename"="lowsponsors.xml", "Header Title String"="Low Sponsor Image List", "Image Information In"=w157) -> ("Image Information Out"=w156:T1)  [unwired: 8 in]
        n123 = local write "Low Sponsor Image List"(w156) -> ()
      }
    }
    n124 = local read "stop"() -> (w152:bool)
  }
  n125 = while {
    tunnel: w1 -> [w159]
    stop <- w158 stop-if-true
    n126 = stacked-sequence {
      tunnel: w159 -> [w160 _]
      frame #0 {
        n127 = Wait on Occurrence(2:w160) -> ()  [unwired: 2 in, 1 out]
      }
      frame #1 {
        n128 = call "ConfigureSounds.vi"() -> ("Sound Cluster"=w176:T3, "output cluster"=w175:T20)  [unwired: 10 in]
        n129 = local write "Sound Cluster"(w176) -> ()
        n130 = Unbundle By Name(w175) -> ("Master Volume"=w174:dbl, "Pre-Primary (s)"=w173:dbl, "Primary (s)"=w172:dbl, "Secondary (s)"=w171:dbl, "Start Sound Path"=w170:path, "Stop Sound Path"=w169:path, "Uh-Oh Sound Path"=w168:path, "Pre-Match Countdown Sound"=w167:path, "Hurry Up Sound"=w166:path, "Start Sound Volume"=w165:dbl, "Stop Sound Volume"=w164:dbl, "Uh-Oh Sound Volume"=w163:dbl, "Pre-Match Coundown Sound Volume"=w162:dbl, "Hurry Up Sound Volume"=w161:dbl)
        n131 = local write "Pre-Match Coundown Sound Volume"(w162) -> ()
        n132 = local write "Pre-Match Countdown Sound"(w167) -> ()
        n133 = local write "Hurry-Up Sound Volume"(w161) -> ()
        n134 = local write "Uh-Oh Sound Volume"(w163) -> ()
        n135 = local write "Start Sound Volume"(w165) -> ()
        n136 = local write "Uh-Oh Sound Path"(w168) -> ()
        n137 = local write "Stop Sound Volume"(w164) -> ()
        n138 = local write "Stop Sound Path"(w169) -> ()
        n139 = local write "Start Sound Path"(w170) -> ()
        n140 = local write "Hurry-Up Sound"(w166) -> ()
        n141 = local write "Master Volume"(w174) -> ()
        n142 = local write "Pre-Primary (s)"(w173) -> ()
        n143 = local write "Secondary (s)"(w171) -> ()
        n144 = local write "Primary (s)"(w172) -> ()
      }
    }
    n145 = local read "stop"() -> (w158:bool)
  }
  n146 = Generate Occurrence() -> (w7:refnum<k4>)
  n147 = while "Button Handler Loop" {
    tunnel: w6 -> [_]
    tunnel: w7 -> [w182]
    tunnel: w5 -> [w181]
    tunnel: w3 -> [w180]
    tunnel: w4 -> [w179]
    tunnel: w2 -> [w178]
    tunnel: w1 -> [w177]
    stop <- w184 stop-if-true
    n148 = event shown="[19] Panel Close?" {
      selector: _ -> [_ _ _ _ _ _ _ _ _ _ _ _ _ _ _ _ _ _ _ _ _ _ _ _ _ _ _ _ _ _ _ _ _ _ _ _ _ _ _ _]
      dyn-events: _ -> [_ _ _ _ _ _ _ _ _ _ _ _ _ _ _ _ _ _ _ _ _ _ _ _ _ _ _ _ _ _ _ _ _ _ _ _ _ _ _ _]
      timeout: 1000 -> [_ _ _ _ _ _ _ _ _ _ _ _ _ _ _ _ _ _ _ _ _ _ _ _ _ _ _ _ _ _ _ _ _ _ _ _ _ _ _ _]
      tunnel: [_ _ _ _ _ _ _ _ _ _ _ _ _ _ _ _ _ _ _ _ _ _ _ _ _ _ _ _ _ _ _ _ _ _ _ _ _ w641 _ _] -> w184
      tunnel: w182 -> [_ _ _ _ _ _ _ _ _ _ _ _ _ _ _ _ _ _ _ _ _ _ w473 _ _ _ _ _ _ _ _ _ _ _ _ _ _ _ _ _]
      tunnel: w181 -> [_ _ _ _ _ _ _ _ _ _ _ _ _ _ _ w370 _ _ _ _ _ _ _ _ _ _ _ _ _ _ _ _ _ _ _ _ _ _ _ _]
      tunnel: w180 -> [_ _ _ _ _ _ _ _ _ _ _ _ _ _ _ _ _ _ _ _ _ w470 _ _ _ _ _ _ _ _ _ _ _ _ _ _ _ _ _ _]
      tunnel: w179 -> [_ _ _ _ _ _ _ _ _ _ _ _ _ _ _ _ _ _ _ _ w467 _ _ _ _ _ _ _ _ _ _ _ _ _ _ _ _ _ _ _]
      tunnel: w178 -> [_ _ _ _ _ _ _ _ _ _ _ _ _ w362 _ _ _ _ _ _ _ _ _ _ _ _ _ _ _ _ _ _ _ _ _ _ _ _ _ _]
      tunnel: w177 -> [_ _ _ _ _ _ _ _ _ _ _ _ _ _ _ _ _ _ _ _ _ _ _ _ _ _ _ w540 _ _ _ _ _ _ _ _ _ _ _ _]
      event Timeout {
        w210 = u16 0 items=["Get All", "Set", "Reset All", "Force Set"] ("Get/Set Mode Selector")
        n149 = event-data() -> ()  [unwired: 1 in, 2 out]
        n150 = local read "Sound Cluster"() -> (w223:T3)
        n151 = Unbundle By Name(w223) -> ("Start"=w222:T27, "Stop"=w216:T27, "Uh-Oh"=w212:T27)
        n152 = Unbundle By Name(w222) -> ("data"=w220:waveform(dbl)[])
        n153 = Unbundle By Name(w216) -> ("data"=w218:waveform(dbl)[])
        n154 = Unbundle By Name(w212) -> ("data"=w213:waveform(dbl)[])
        n155 = Not Equal?(x=w220, y=waveform(dbl)[] [] ("data")) -> (x != y?=→"Start Sound Indicator":bool)
        n156 = Not Equal?(x=w218, y=waveform(dbl)[] [] ("data")) -> (x != y?=→"Stop Sound Indicator":bool)
        n157 = Not Equal?(x=w213, y=waveform(dbl)[] [] ("data")) -> (x != y?=→"Uh-Oh Sound Indicator":bool)
        n158 = local read "Schedule To Show"() -> (w228:enum16{"Practice", "Ranking"})
        n159 = call "Current Match Control.vi"("Mode"=T15."Get") -> ("Current Phase"=w198:enum16{"Practice", "Ranking"})  [unwired: 9 in, 1 out]
        n160 = Equal?(x=w228, y=w198) -> (x = y?=w227:bool)
        n161 = call "ScoreControl.vi"("Get/Set Mode Selector"=w210) -> ("Scores"=w203:T9)  [unwired: 13 in, 1 out]
        "Score Data" <- w203
        n162 = Not Equal?(x=w203, y=T9 []) -> (x != y?=→"Scores Exist":bool)
        n163 = Array Size(array=w203) -> (size(s)=→"Number of Scores":i32)
        n164 = case shown="True" w227 {
          tunnel: [-1 ("Schedule") w245] -> w226
          frame False {
          }
          frame True {
            n165 = call "Current Match Control.vi"("Mode"=T15."Get") -> ("Current Match"=w246:u16)  [unwired: 9 in, 1 out]
            n166 = Decrement(x=w246) -> (x-1=w245:u16)
          }
        }
        n167 = call "Team Data Control.vi"("Mode"=T13."Get Teams") -> ("Team Array Out"=w197:T7[])  [unwired: 10 in]
        n168 = Not Equal?(x=w197, y=T7[] []) -> (x != y?=→"Teams Exist":bool)
        n169 = call "IPRegistry.vi"("Action"=enum16{"Flush All", "Lookup", "Add"}."Lookup") -> ("Users"=w187:string[])  [unwired: 9 in, 1 out]
        n170 = Array Size(array=w187) -> (size(s)=w186:i32)
        n171 = call "Build Text"("num"=w186) -> ("Result"=w185:string)  [unwired: 13 in, 1 out]
        n172 = local write "Team Info"(w197) -> ()
        n173 = local write "Schedule"(w226) -> ()
        n174 = local write "Users String"(w185) -> ()
        n175 = Array Size(array=w197) -> (size(s)=→"Number of Teams":i32)
        n176 = call "Get Team Ranking.vi"("Needed Validations"="Needed Validations") -> ("Ranked Teams"=w190:T28)  [unwired: 10 in]
        n177 = for {
          tunnel: w190 -> [w238] mode=indexing
          tunnel: [w232] -> w200 mode=indexing
          n178 = Unbundle By Name(w238) -> ("Team Number"=w237:u16, "Team Name"=w235:string, "Highest Score"=w234:dbl, "Scores"=w231:cluster{"Score":dbl, "Round":u16}[])
          n179 = Number To Decimal String(number=w237) -> (decimal integer string=w236:string)  [unwired: 1 in]
          n180 = Number To Fractional String(number=w234, precision (6)=i16 0) -> (F-format string=w233:string)  [unwired: 2 in]
          n181 = for {
            tunnel: w231 -> [w242] mode=indexing
            tunnel: [w240] -> w230 mode=indexing
            n182 = Unbundle By Name(w242) -> ("Score"=w241:dbl)
            n183 = Number To Fractional String(number=w241, precision (6)=i16 0) -> (F-format string=w240:string)  [unwired: 2 in]
          }
          n184 = Build Array (concatenate)(w236, w235, w233, w230) -> (w232:string[])
        }
        "Team Rankings" <- w200
        n185 = call "Calculate Team Ranking Positions.vi"("Ranked Teams in"=w190) -> ("Rankings"=w189:string[])  [unwired: 9 in, 1 out]
        n186 = property on="Team Rankings" class="Tbl (strict)"("Row Headers[]"=w189) -> ()  [unwired: 2 in, 2 out]
        n187 = String To IP() -> (0:w225:u32)  [unwired: 1 in]
        n188 = local read "Port"() -> (w193:string)
        n189 = IP To String(1:TRUE ("dot notation? (F)"), 2:w225) -> (0:w195:string)
        "Current IP" <- w195
        n190 = Concatenate Strings("http://", w195, ":", w193, "/FLL") -> (→"Web Interface Location":string)
      }
      event "Start New Game Button": Value Change {
        n191 = event-data() -> ("CtlRef"=w247:refnum<vi>)  [unwired: 1 in, 5 out]
        n192 = stacked-sequence {
          tunnel: w247 -> [_ w250]
          frame #0 {
            n193 = local write "Startup Navigation Tab Control"(enum32{"Start", "New", "Done"}."New" ("Startup Navigation Tab Control")) -> ()
          }
          frame #1 {
            n194 = property class="Bool (strict)"(reference=w250, "Value"=FALSE) -> ()  [unwired: 1 in, 2 out]
          }
        }
      }
      event "Load Schedule Button": Value Change {
        n195 = event-data() -> ("CtlRef"=w261:refnum<vi>)  [unwired: 1 in, 5 out]
        n196 = local read "Schedule File Path"() -> (w255:path)
        n197 = property class="Bool (strict)"(reference=w261, "Value"=FALSE) -> ()  [unwired: 1 in, 2 out]
        n198 = call "File Dialog2"("start path"=w255, "prompt"="Load Bryan Lee Tournament .csv Export File", "button label"="Load Schedule", "pattern (all files)"="*.csv", "pattern label"="Comma Separated Values") -> ("selected path"=w251:path, "exists"=w252:bool, "cancelled"=w253:bool)  [unwired: 7 in, 1 out]
        n199 = Compound Arithmetic op=AND(invert w253, w252) -> (w254:bool)
        n200 = case shown="True" w254 {
          tunnel: w251 -> [_ w262]
          frame False {
          }
          frame True {
            n201 = local write "Schedule File Path"(w262) -> ()
            n202 = flat-sequence {
              tunnel: [w266] -> w264
              tunnel: w262 -> [w265]
              tunnel: w264 -> [w302]
              tunnel: [w301] -> w263
              tunnel: w263 -> [w322]
              frame #0 {
                n203 = call "ReadScheduleFile.vi"("Enum"=enum16{"Load", "Get"}."Load", "Team Info / Schedule File"=w265) -> ("error out"=w267:errorcluster, "PracticeMatches"=w271:string[][], "RankingMatches"=w272:string[][], "Team Information"=w273:cluster{string, "[0]":string, "[1]":string}[], "Table Names"=w268:string[], "Practice Match Times"=w269:string[][], "Ranking Match Times"=w270:string[][])  [unwired: 2 in, 1 out]
                n204 = case shown="No Error" w267 {
                  selector: w267 -> [w275 w300]
                  tunnel: w273 -> [w287 _]
                  tunnel: w272 -> [w286 _]
                  tunnel: w271 -> [w285 _]
                  tunnel: w270 -> [w281 _]
                  tunnel: w269 -> [w280 _]
                  tunnel: w268 -> [w276 _]
                  tunnel: [w275 w300] -> w266
                  frame No Error {
                    n205 = call "Team Data Control.vi"("Mode"=T24."Clear All Teams") -> ("Team Array Out"=w288:T7[])  [unwired: 10 in]
                    n206 = for {
                      tunnel: w287 -> [w296] mode=indexing
                      tunnel: w288 -> [_]
                      tunnel: [w290] -> w278
                      n207 = Unbundle(w296) -> (w291:string, "[0]"=w293:string, "[1]"=w295:string)
                      n208 = Decimal String To Number(string=w293, default (0L)=u16 0) -> (number=w294:u16)  [unwired: 1 in, 1 out]
                      n209 = Bundle By Name(cluster=T7 {"Both"="", "Name"="", "GUID"=0, "Number"=0} ("Team Data"), "Both"=w291, "Name"=w295, "Number"=w294) -> (w297:T7)
                      n210 = call "Team Data Control.vi"("Team Data To Add/Change"=w297, "Mode"=T24."Add Team") -> ("Team Array Out"=w290:T7[])  [unwired: 9 in]
                    }
                    n211 = local write "Table Names"(w276) -> ()
                    n212 = Bundle By Name(cluster=T23 {"Practice Matches"=[], "Ranking Matches"=[], "Table Names"=[], "Ranking Match Times"=[], "Practice Match Times"=[]} ("Schedule Data"), "Ranking Matches"=w286, "Practice Matches"=w285, "Table Names"=w276, "Ranking Match Times"=w281, "Practice Match Times"=w280) -> (w282:T23)
                    n213 = call "Schedule Control.vi"("Schedule Data"=w282, "Mode"=enum16{"Get", "Set"}."Set") -> ()  [unwired: 9 in, 1 out]
                    n214 = local read "Team Data File Path"() -> (w277:path)
                    n215 = Flatten To XML(anything=w278) -> (xml string=w279:string)
                    n216 = call-poly <vilib>:"Write to XML File.vi"("XML Input"=w279, "XML File Path"=w277) -> ()  [unwired: 7 in, 3 out]
                  }
                  frame Error {
                  }
                }
              }
              frame #1 {
                n217 = case shown="No Error" w302 {
                  selector: w302 -> [w303 w321]
                  tunnel: [w303 w321] -> w301
                  frame No Error {
                    n218 = local read "Schedule To Show"() -> (w304:enum16{"Practice", "Ranking"})
                    n219 = call "Schedule Control.vi"("Mode"=enum16{"Get", "Set"}."Get") -> ("Schedule Data Out"=w313:T23)  [unwired: 10 in]
                    n220 = case shown="\"Practice\", Default" w304 {
                      tunnel: w313 -> [w318 w320]
                      tunnel: [w317 w319] -> w305
                      frame "Practice", Default {
                        n221 = Unbundle By Name(w318) -> ("Practice Matches"=w317:string[][])
                      }
                      frame "Ranking" {
                        n222 = Unbundle By Name(w320) -> ("Ranking Matches"=w319:string[][])
                      }
                    }
                    n223 = Unbundle By Name(w313) -> ("Table Names"=w314:string[])
                    n224 = Array Subset(array=w305, index (col)=1 ("index")) -> (w311:string[][])  [unwired: 3 in]
                    n225 = Array Subset(array=w305, index (col)=0 ("index"), length (col)=1 ("length")) -> (w307:string[][])  [unwired: 2 in]
                    n226 = for {
                      tunnel: w307 -> [w316] mode=indexing
                      tunnel: [w315] -> w310 mode=indexing
                      n227 = Index Array(array=w316) -> (element=w315:string)  [unwired: 1 in]
                    }
                    n228 = property on="Schedule" class="MCListbox (strict)"("ItemNames"=w311) -> ()  [unwired: 2 in, 2 out]
                    n229 = property on="Schedule" class="MCListbox (strict)"("ColHdrString"=w314, "RowHdrs[]"=w310) -> ()  [unwired: 2 in, 2 out]
                  }
                  frame Error {
                  }
                }
              }
              frame #2 {
                n230 = case shown="No Error" w322 {
                  frame No Error {
                    n231 = stacked-sequence {
                      frame #0 {
                        n232 = local write "Startup Navigation Tab Control"(enum32{"Start", "New", "Done"}."Done" ("Startup Navigation Tab Control")) -> ()
                        n233 = call "Display Message to User"() -> ()  [unwired: 10 in, 2 out]
                      }
                      frame #1 {
                        w324 = T21."Enabled" ("Disabled")
                        n234 = property on="Local Entry Button" class="Bool (strict)"("DisabledEnum"=w324) -> ()  [unwired: 2 in, 2 out]
                        n235 = property on="System Monitor Button" class="Bool (strict)"("DisabledEnum"=w324) -> ()  [unwired: 2 in, 2 out]
                        n236 = property on="View Rankings Button" class="Bool (strict)"("DisabledEnum"=w324) -> ()  [unwired: 2 in, 2 out]
                        n237 = property on="Launch Score Entry" class="Bool (strict)"("DisabledEnum"=w324) -> ()  [unwired: 2 in, 2 out]
                        n238 = property on="Go to Timekeeper Button" class="Bool (strict)"("DisabledEnum"=w324) -> ()  [unwired: 2 in, 2 out]
                        n239 = property on="Settings Button" class="Bool (strict)"("DisabledEnum"=w324) -> ()  [unwired: 2 in, 2 out]
                        n240 = property on="Profile Button" class="Bool (strict)"("DisabledEnum"=w324) -> ()  [unwired: 2 in, 2 out]
                      }
                    }
                  }
                  frame Error {
                    n241 = call "Display Message to User2"() -> ()  [unwired: 10 in, 2 out]
                  }
                }
              }
            }
          }
        }
      }
      event "New Game Back Button": Value Change {
        n242 = event-data() -> ("CtlRef"=w327:refnum<vi>, "OldVal"=w326:bool)  [unwired: 1 in, 4 out]
        n243 = property class="Bool (strict)"(reference=w327, "Value"=w326) -> ()  [unwired: 1 in, 2 out]
        n244 = local write "Startup Navigation Tab Control"(enum32{"Start", "New", "Done"}."Start" ("Startup Navigation Tab Control")) -> ()
      }
      event "Launch Web Server Button": Value Change {
        n245 = event-data() -> ("CtlRef"=w330:refnum<vi>, "OldVal"=w329:bool)  [unwired: 1 in, 4 out]
        n246 = property class="Bool (strict)"(reference=w330, "Value"=w329) -> ()  [unwired: 1 in, 2 out]
        n247 = local read "Web Interface Location"() -> (w328:string)
        n248 = call-poly <vilib>:"Open URL in Default Browser.vi"("URL"=w328) -> ()  [unwired: 5 in, 2 out]
      }
      event "Settings Button": Value Change {
        n249 = event-data() -> ("CtlRef"=w332:refnum<vi>, "OldVal"=w331:bool)  [unwired: 1 in, 4 out]
        n250 = property class="Bool (strict)"(reference=w332, "Value"=w331) -> ()  [unwired: 1 in, 2 out]
        n251 = local write "Tab Control"(T25."System Control" ("Tab Control")) -> ()
      }
      event "Profile Button": Value Change {
        n252 = event-data() -> ("CtlRef"=w336:refnum<vi>, "OldVal"=w335:bool)  [unwired: 1 in, 4 out]
        n253 = property class="Bool (strict)"(reference=w336, "Value"=w335) -> ()  [unwired: 1 in, 2 out]
        n254 = local write "Tab Control"(T5."Profiles" ("Tab Control")) -> ()
      }
      event "Go to Timekeeper Button": Value Change {
        n255 = event-data() -> ("CtlRef"=w340:refnum<vi>, "OldVal"=w339:bool)  [unwired: 1 in, 4 out]
        n256 = property class="Bool (strict)"(reference=w340, "Value"=w339) -> ()  [unwired: 1 in, 2 out]
        n257 = local write "Splash Page Main Tab Control"(T17."Timekeeper" ("Splash Page Main Tab Control")) -> ()
        n258 = local write "Tab Control"(T5."Splash" ("Tab Control")) -> ()
      }
      event "View Rankings Button": Value Change {
        n259 = event-data() -> ("CtlRef"=w343:refnum<vi>, "OldVal"=w342:bool)  [unwired: 1 in, 4 out]
        n260 = property class="Bool (strict)"(reference=w343, "Value"=w342) -> ()  [unwired: 1 in, 2 out]
        n261 = local write "Tab Control"(T5."Splash" ("Tab Control")) -> ()
        n262 = local write "Splash Page Main Tab Control"(T17."Rankings" ("Splash Page Main Tab Control")) -> ()
      }
      event "System Monitor Button": Value Change {
        n263 = event-data() -> ("CtlRef"=w345:refnum<vi>, "OldVal"=w346:bool)  [unwired: 1 in, 4 out]
        n264 = property class="Bool (strict)"(reference=w345, "Value"=w346) -> ()  [unwired: 1 in, 2 out]
        n265 = local write "Tab Control"(T25."System Monitor" ("Tab Control")) -> ()
      }
      event "Home Button": Value Change {
        n266 = event-data() -> ("CtlRef"=w350:refnum<vi>, "OldVal"=w351:bool)  [unwired: 1 in, 4 out]
        n267 = property class="Bool (strict)"(reference=w350, "Value"=w351) -> ()  [unwired: 1 in, 2 out]
        n268 = local write "Splash Page Main Tab Control"(T17."Main Splash Instructions" ("Splash Page Main Tab Control")) -> ()
        n269 = local write "Tab Control"(T5."Splash" ("Tab Control")) -> ()
      }
      event "Timer Start": Value Change {
        n270 = event-data() -> ("CtlRef"=w356:refnum<vi>)  [unwired: 1 in, 1 out]
        n271 = property class="Bool (strict)"(reference=w356, "Value"=FALSE) -> ()  [unwired: 1 in, 2 out]
        n272 = call "Timer Running Control.vi"("Enum"=T14."Start Timer") -> ()  [unwired: 10 in, 1 out]
        n273 = call "Log Message.vi"("Message"="Local user started the timer.", "Log"=enum16{"Error Log", "Timer Log", "Scoring Log"}."Timer Log") -> ()  [unwired: 10 in]
      }
      event "Timer Stop": Value Change {
        n274 = event-data() -> ("CtlRef"=w361:refnum<vi>)  [unwired: 1 in, 3 out]
        n275 = property class="Bool (strict)"(reference=w361, "Value"=FALSE) -> ()  [unwired: 1 in, 2 out]
        n276 = call "Timer Running Control.vi"("Enum"=T14."Stop Timer") -> ()  [unwired: 10 in, 1 out]
        n277 = call "Log Message.vi"("Message"="Local user stopped the timer.", "Log"=enum16{"Error Log", "Timer Log", "Scoring Log"}."Timer Log") -> ()  [unwired: 10 in]
      }
      event "Create/Edit Team List", "Edit Team Information Button": Value Change {
        n278 = event-data() -> ("CtlRef"=w364:refnum<vi>, "OldVal"=w363:bool)  [unwired: 1 in, 4 out]
        n279 = Set Occurrence(w362) -> ()
        n280 = property class="Bool (strict)"(reference=w364, "Value"=w363) -> ()  [unwired: 1 in, 2 out]
      }
      event "Score Entry", "Launch Score Entry": Value Change {
        n281 = event-data() -> ("CtlRef"=w369:refnum<vi>)  [unwired: 1 in, 5 out]
        n282 = property class="Bool (strict)"(reference=w369, "Value"=FALSE) -> ()  [unwired: 1 in, 2 out]
        n283 = local read "Web Interface Location"() -> (w366:string)
        n284 = Concatenate Strings(w366, "/ScoreEntry" ("URL")) -> (w367:string)
        n285 = call-poly <vilib>:"Open URL in Default Browser.vi"("URL"=w367) -> ()  [unwired: 5 in, 2 out]
      }
      event "Config Top Sponsors Button": Value Change {
        n286 = event-data() -> ("CtlRef"=w372:refnum<vi>, "OldVal"=w371:bool)  [unwired: 1 in, 4 out]
        n287 = Set Occurrence(w370) -> ()
        n288 = property class="Bool (strict)"(reference=w372, "Value"=w371) -> ()  [unwired: 1 in, 2 out]
      }
      event "Display Screen Title": Value Change {
        n289 = event-data() -> ("NewVal"=w375:string)  [unwired: 1 in, 5 out]
        n290 = call "GetSetProfileInfo.vi"("Parameter"=enum16{"Logo Path", "Logo", "Title"}."Title", "Get/Set State"=enum16{"Get", "Set", "Load"}."Set", "Title"=w375) -> ()  [unwired: 4 in, 5 out]
      }
      event "Main Logo Image (129x462)": Value Change {
        n291 = event-data() -> ("NewVal"=w382:path)  [unwired: 1 in, 5 out]
        n292 = call "GetSetProfileInfo.vi"("Parameter"=enum16{"Logo Path", "Logo", "Title"}."Logo Path", "Get/Set State"=enum16{"Get", "Set", "Load"}."Set", "Logo Path In"=w382) -> ("Logo Path Out"=w381:path)  [unwired: 4 in, 4 out]
        n293 = call "Score Display - Load Image (LV).vi"("path to image file"=w381) -> ("image data"=w378:T22)
        n294 = call "GetSetProfileInfo.vi"("Parameter"=enum16{"Logo Path", "Logo", "Title"}."Logo", "Get/Set State"=enum16{"Get", "Set", "Load"}."Set", "image data"=w378) -> ("image data out"=w376:T22)  [unwired: 4 in, 4 out]
        n295 = control-ref of="Preview"() -> (w377:refnum<vi>)
        n296 = call "Score Display - Display Image (LV).vi"("image data"=w376, "Picture Reference"=w377) -> ()  [unwired: 2 in]
      }
      event "Rounds to Show": Value Change {
        n297 = event-data() -> ("NewVal"=w386:u16)  [unwired: 1 in, 5 out]
        n298 = call "GetSetProfileInfo.vi"("Parameter"=enum16{"Logo Path", "Logo", "Title", "Rounds"}."Rounds", "Get/Set State"=enum16{"Get", "Set", "Load"}."Set", "Rounds To Show In"=w386) -> ()  [unwired: 4 in, 5 out]
      }
      event Panel Close? {
        w390 = "\r\n"
        n299 = event-data() -> ()  [unwired: 1 in, 4 out]
        n300 = Concatenate Strings("Would you like for me to make a backup of all files " ("message"), w390, "(including a human-readable CSV) in a ZIP file " ("message"), w390, "(maybe for USB Backup or so) before you go?" ("message")) -> (w388:string)
        n301 = call <vilib>:"Three Button Dialog.vi"("Window Title (\"\")"="Want to Backup your Scores and Files?" ("Window Title (\"\")"), "message"=w388) -> ("Which Button?"=w394:T29)  [unwired: 9 in]
        n302 = case shown="\"Left Button\", Default" w394 {
          tunnel: [w397 TRUE FALSE FALSE] -> w393
          frame "Left Button", Default {
            # "YES - Save a copy."
            n303 = call "File Dialog3"("prompt"="Select Backup File Location", "button label"="SAVE", "pattern (all files)"="*.zip", "pattern label"="ZIP") -> ("selected path"=w400:path, "cancelled"=w399:bool)  [unwired: 8 in, 2 out]
            n304 = call <vilib>:"New Zip File.vi"("confirm overwrite? (F)"=FALSE, "target"=w400) -> ("zip file out"=w404:i64)  [unwired: 3 in, 2 out]
            n305 = case shown="False" w399 {
              tunnel: w404 -> [w407 _]
              tunnel: [TRUE FALSE] -> w397
              frame False {
                n306 = stacked-sequence {
                  tunnel: w407 -> [_ w448]
                  frame #0 {
                    w415 = T19 7 items=["User Home"=0, "User Desktop"=1, "User Documents"=2, "User Application Data"=3, "User Preferences"=4, "User Temporary"=5, "Public Documents"=6, "Public Application Data"=7, "Public Preferences"=8, "Public Cache"=13, "System Core Libraries"=9, "System Installed Libraries"=10, "Application Files"=11, "Boot Volume Root"=12] ("system directory type")
                    n307 = call <vilib>:"Get System Directory.vi"("system directory type"=w415) -> ("system directory"=w414:path)  [unwired: 10 in]
                    n308 = Build Path(base path=w414, name or relative path="FLL\\Data\\scoresfile.csv") -> (appended path=w412:path)
                    n309 = Open/Create/Replace File(file path (use dialog)=w412, operation (0:open)=T26."replace or create", access (0:read/write)=enum16{"read/write", "read-only", "write-only"}."write-only") -> (refnum out=w410:refnum<file>, error out=w411:errorcluster)  [unwired: 3 in, 1 out]
                    n310 = case shown="No Error" w411 {
                      tunnel: w411 -> [w421 _]
                      tunnel: w410 -> [w422 _]
                      tunnel: "Rank,Team Number,Team Name,Highest Score,Match1,Match2,Match3,Match4 " -> [w419 _]
                      frame No Error {
                        n311 = property on="Team Rankings" class="Tbl (strict)"() -> ("Row Headers[]"=w430:string[])  [unwired: 2 in, 2 out]
                        n312 = local read "Team Rankings"() -> (w429:string[][])
                        n313 = for {
                          tunnel: w430 -> [w436] mode=indexing
                          tunnel: w429 -> [w433] mode=indexing
                          tunnel: "" -> [w434]
                          tunnel: [w431] -> w425 mode=indexing
                          n314 = for {
                            shift-right: [w437] -> w432
                            shift-left: w434 -> [w440]
                            tunnel: w433 -> [w438] mode=indexing
                            n315 = Concatenate Strings(w440, w438, "," ("string")) -> (w437:string)
                          }
                          n316 = Concatenate Strings(w436, "," ("string"), w432) -> (w431:string)
                        }
                        n317 = Concatenate Strings(w419, "\r\n") -> (w420:string)
                        n318 = Write to Text File(file (use dialog)=w422, text=w420, error in=w421) -> (refnum out=w424:refnum<file>, error out=w423:errorcluster)  [unwired: 1 in, 1 out]
                        n319 = Write to Text File(file (use dialog)=w424, text=w425, error in=w423) -> (refnum out=w426:refnum<file>, error out=w427:errorcluster)  [unwired: 1 in, 1 out]
                        n320 = Close File(refnum=w426, error in=w427) -> (error out=w417:errorcluster)  [unwired: 1 out]
                        n321 = case shown="No Error" w417 {
                          frame No Error {
                          }
                          frame Error {
                            n322 = call "Display Message to User8"() -> ()  [unwired: 10 in, 2 out]
                          }
                        }
                      }
                      frame Error {
                        n323 = call "Display Message to User9"() -> ()  [unwired: 10 in, 2 out]
                      }
                    }
                  }
                  frame #1 {
                    w452 = T19 7 items=["User Home"=0, "User Desktop"=1, "User Documents"=2, "User Application Data"=3, "User Preferences"=4, "User Temporary"=5, "Public Documents"=6, "Public Application Data"=7, "Public Preferences"=8, "Public Cache"=13, "System Core Libraries"=9, "System Installed Libraries"=10, "Application Files"=11, "Boot Volume Root"=12] ("system directory type")
                    n324 = call <vilib>:"Get System Directory.vi"("system directory type"=w452) -> ("system directory"=w451:path)  [unwired: 10 in]
                    n325 = Build Path(base path=w451, name or relative path="FLL") -> (appended path=w449:path)
                    n326 = call <vilib>:"Recursive File List.vi"("Continue Recursing on Error? (F)"=TRUE, "Treat LLBs as Folders?"=FALSE, "Folder Path"=w449) -> ("All Files in Dir"=w447:path[])  [unwired: 4 in, 4 out]
                    n327 = for {
                      tunnel: w448 -> [w462]
                      tunnel: w447 -> [w460] mode=indexing
                      tunnel: [w461] -> w445
                      n328 = Strip Path(path=w460) -> (stripped path=w459:path, name=w458:string)
                      n329 = Strip Path(path=w459) -> (name=w456:string)  [unwired: 1 out]
                      n330 = String To Path(string=w456) -> (path=w455:path)
                      n331 = Build Path(base path=w455, name or relative path=w458) -> (appended path=w457:path)
                      n332 = call <vilib>:"Add File to Zip.vi"("destination path in zip"=w457, "source file path"=w460, "zip file in"=w462) -> ("zip file out"=w461:i64)  [unwired: 7 in, 1 out]
                    }
                    n333 = local read "Schedule File Path"() -> (w443:path)
                    n334 = Strip Path(path=w443) -> (name=w442:string)  [unwired: 1 out]
                    n335 = String To Path(string=w442) -> (path=w441:path)
                    n336 = call <vilib>:"Add File to Zip.vi"("destination path in zip"=w441, "source file path"=w443, "zip file in"=w445) -> ("zip file out"=w444:i64)  [unwired: 7 in, 1 out]
                    n337 = call <vilib>:"Close Zip File.vi"("zip file in"=w444) -> ("error out"=w446:errorcluster)  [unwired: 6 in]
                    n338 = call <vilib>:"Simple Error Handler.vi"("error in (no error)"=w446) -> ()  [unwired: 4 in, 5 out]
                  }
                }
              }
              frame True {
              }
            }
          }
          frame "Center Button" {
            # "NO - don't want to save a backup (piss off!)"
          }
          frame "Right Button" {
            # "CANCEL - do not want to exit"
          }
          frame "Window Close" {
            # "Window Close - Do not allow an exit"
          }
        }
        n339 = Not(x=w393) -> (.not. x?=w396:bool)
        n340 = event-data("Discard?"=w396) -> ()  [unwired: 1 in, 1 out]
      }
      event "Config Mid Sponsors Button": Value Change {
        n341 = event-data() -> ("CtlRef"=w469:refnum<vi>, "OldVal"=w468:bool)  [unwired: 1 in, 4 out]
        n342 = Set Occurrence(w467) -> ()
        n343 = property class="Bool (strict)"(reference=w469, "Value"=w468) -> ()  [unwired: 1 in, 2 out]
      }
      event "Config Low Sponsors Button": Value Change {
        n344 = event-data() -> ("CtlRef"=w472:refnum<vi>, "OldVal"=w471:bool)  [unwired: 1 in, 4 out]
        n345 = Set Occurrence(w470) -> ()
        n346 = property class="Bool (strict)"(reference=w472, "Value"=w471) -> ()  [unwired: 1 in, 2 out]
      }
      event "Write Score Data To Human-Readable CSV File": Value Change {
        # "Set Occurrence for creating human-readable CSV file."
        n347 = event-data() -> ("CtlRef"=w474:refnum<vi>)  [unwired: 1 in, 1 out]
        n348 = Set Occurrence(w473) -> ()
        n349 = flat-sequence {
          tunnel: w474 -> [w476]
          frame #0 {
            n350 = property class="Bool (strict)"(reference=w476, "Value"=FALSE) -> ()  [unwired: 1 in, 2 out]
          }
        }
      }
      event "Replace Current Score Data\nFrom File": Value Change {
        n351 = event-data() -> ("CtlRef"=w480:refnum<vi>)  [unwired: 1 in, 5 out]
        n352 = property class="Bool (strict)"(reference=w480, "Value"=FALSE) -> ()  [unwired: 1 in, 2 out]
        n353 = Two Button Dialog(message="This will permenantly replace the current scoring data with the contents of the file. Are you really bloody sure?") -> (T button?=w477:bool)  [unwired: 2 in]
        n354 = case shown="True" w477 {
          frame False {
          }
          frame True {
            n355 = case shown="\"LabVIEW Flat XML\"" "Input File Type" {
              tunnel: "Score File Path (Read)" -> [w483 w488 w490]
              frame "Human Readable XML", Default {
                n356 = call "Read Score Data From File.vi"("XML File Path"=w483) -> ()  [unwired: 10 in, 1 out]
              }
              frame "LabVIEW Flat XML" {
                w485 = u16 4 items=["Get All", "Set", "Reset All", "Force Set", "Force Set All"] ("Get/Set Mode Selector")
                n357 = call-poly <vilib>:"Read From XML File.vi"("XML File Path"=w488) -> ("error out"=w487:errorcluster, "XML Elements"=w489:string)  [unwired: 8 in, 1 out]
                n358 = Unflatten From XML(xml string=w489, type=T9 [] ("Scores"), error in (no error)=w487) -> (value=w484:T9)  [unwired: 1 out]
                n359 = call "ScoreControl.vi"("Get/Set Mode Selector"=w485, "All Scores"=w484) -> ()  [unwired: 12 in, 2 out]
              }
              frame "Build From Score Files" {
                n360 = call "Rebuild Score Data From Files.vi"("Score Files Directory"=w490) -> ()  [unwired: 11 in]
              }
            }
          }
        }
      }
      event "Schedule To Show": Value Change {
        n361 = event-data() -> ("NewVal"=w501:enum16{"Practice", "Ranking"})  [unwired: 1 in, 5 out]
        n362 = call "Schedule Control.vi"("Mode"=enum16{"Get", "Set"}."Get") -> ("Schedule Data Out"=w492:T23)  [unwired: 10 in]
        n363 = case shown="\"Practice\", Default" w501 {
          tunnel: w492 -> [w505 w507]
          tunnel: [w504 w506] -> w500
          frame "Practice", Default {
            n364 = Unbundle By Name(w505) -> ("Practice Matches"=w504:string[][])
          }
          frame "Ranking" {
            n365 = Unbundle By Name(w507) -> ("Ranking Matches"=w506:string[][])
          }
        }
        n366 = Unbundle By Name(w492) -> ("Table Names"=w491:string[])
        n367 = Array Subset(array=w500, index (col)=1 ("index")) -> (w494:string[][])  [unwired: 3 in]
        n368 = Array Subset(array=w500, index (col)=0 ("index"), length (col)=1 ("length")) -> (w498:string[][])  [unwired: 2 in]
        n369 = for {
          tunnel: w498 -> [w503] mode=indexing
          tunnel: [w502] -> w495 mode=indexing
          n370 = Index Array(array=w503) -> (element=w502:string)  [unwired: 1 in]
        }
        n371 = property on="Schedule" class="MCListbox (strict)"("ItemNames"=w494) -> ()  [unwired: 2 in, 2 out]
        n372 = property on="Schedule" class="MCListbox (strict)"("ColHdrString"=w491, "RowHdrs[]"=w495) -> ()  [unwired: 2 in, 2 out]
      }
      event Value Change {
        n373 = event-data() -> ("OldVal"=w514:T6, "NewVal"=w513:T6)  [unwired: 1 in, 4 out]
        n374 = for {
          tunnel: w514 -> [w523] mode=indexing
          tunnel: w513 -> [w521] mode=indexing
          tunnel: [w522] -> w512
          tunnel: [w521] -> w511
          stop <- w522 stop-if-true
          n375 = Not Equal?(x=w523, y=w521) -> (x != y?=w522:bool)
        }
        n376 = case shown="False" w512 {
          tunnel: w511 -> [_ w519]
          tunnel: [w515 w517] -> w508
          frame False {
            n377 = call "Team Data Control.vi"("Mode"=T13."Get Teams") -> ("Team Array Out"=w515:T7[])  [unwired: 10 in]
          }
          frame True {
            n378 = Unbundle By Name(w519) -> ("GUID"=w518:u16)
            n379 = call "Team Data Control.vi"("GUID To Modify"=w518, "Team Data To Add/Change"=w519, "Mode"=T13."Modify Team") -> ("Team Array Out"=w517:T7[])  [unwired: 8 in]
          }
        }
        n380 = local read "Team Data File Path"() -> (w509:path)
        n381 = Flatten To XML(anything=w508) -> (xml string=w510:string)
        n382 = call-poly <vilib>:"Write to XML File.vi"("XML Input"=w510, "XML File Path"=w509) -> ()  [unwired: 7 in, 3 out]
      }
      event "Delete Team": Value Change {
        n383 = event-data() -> ("CtlRef"=w524:refnum<vi>)  [unwired: 1 in]
        n384 = property class="Bool (strict)"(reference=w524, "Value"=FALSE) -> ()  [unwired: 1 in, 2 out]
        n385 = property on="Team Info" class="Arr (strict)"() -> ("Index Values"=w537:u32[], "Value"=w535:T6)  [unwired: 2 in, 2 out]
        n386 = Index Array(array=w537, index=0) -> (element=w534:u32)
        n387 = Index Array(array=w535, index=w534) -> (element=w533:T7)
        n388 = Unbundle By Name(w533) -> ("Number"=w532:u16, "GUID"=w526:u16)
        n389 = Number To Decimal String(number=w532) -> (decimal integer string=w529:string)  [unwired: 1 in]
        n390 = Concatenate Strings("Are you really sure you want to delete team " ("string"), w529, "?" ("string")) -> (w527:string)
        n391 = Two Button Dialog(message=w527) -> (T button?=w531:bool)  [unwired: 2 in]
        n392 = case shown="True" w531 {
          tunnel: w526 -> [_ w538]
          frame False {
          }
          frame True {
            n393 = call "Team Data Control.vi"("GUID To Modify"=w538, "Mode"=T13."Delete Team") -> ()  [unwired: 9 in, 1 out]
          }
        }
      }
      event "Configure Sounds Button": Value Change {
        n394 = event-data() -> ()  [unwired: 1 in, 6 out]
        n395 = Set Occurrence(w540) -> ()
      }
      event "Score Entry Access Password": Value Change {
        n396 = event-data() -> ("NewVal"=w541:string)  [unwired: 1 in, 5 out]
        n397 = call "password.vi"("Action"=enum16{"Compare", "Set"}."Set", "password"=w541) -> ()  [unwired: 9 in, 1 out]
      }
      event "Clear Access List Button": Value Change {
        n398 = event-data() -> ()  [unwired: 1 in, 6 out]
        n399 = call "IPRegistry.vi"("Action"=enum16{"Flush All", "Lookup", "Add"}."Flush All") -> ()  [unwired: 9 in, 2 out]
      }
      event "Previous Match": Value Change {
        n400 = event-data() -> ("CtlRef"=w546:refnum<vi>)  [unwired: 1 in, 1 out]
        n401 = property class="Bool (strict)"(reference=w546, "Value"=FALSE) -> ()  [unwired: 1 in, 2 out]
        n402 = call "Current Match Control.vi"("Mode"=T15."Decrement") -> ("Current Match"=w545:u16)  [unwired: 9 in, 1 out]
        n403 = local write "Current Match"(w545) -> ()
      }
      event "Next Match": Value Change {
        n404 = event-data() -> ("CtlRef"=w550:refnum<vi>)  [unwired: 1 in, 5 out]
        n405 = property class="Bool (strict)"(reference=w550, "Value"=FALSE) -> ()  [unwired: 1 in, 2 out]
        n406 = call "Current Match Control.vi"("Mode"=T15."Increment") -> ("Current Match"=w549:u16)  [unwired: 9 in, 1 out]
        n407 = local write "Current Match"(w549) -> ()
      }
      event "PH 2": Value Change {
        n408 = event-data() -> ("CtlRef"=w554:refnum<vi>)  [unwired: 1 in, 5 out]
        n409 = property class="Bool (strict)"(reference=w554, "Value"=FALSE) -> ()  [unwired: 1 in, 2 out]
        n410 = call "styles.css.vi"("Web"=FALSE, "Mode"=enum16{"G", "S", "T"}."T") -> ("Boolean 2"=w552:bool)  [unwired: 9 in]
        "PH" <- w552
        n411 = property on="PH" class="Bool (strict)"("Visible"=w552) -> ()  [unwired: 2 in, 2 out]
      }
      event "Current Phase": Value Change {
        n412 = event-data() -> ("NewVal"=w557:enum16{"Practice", "Ranking"})  [unwired: 1 in, 5 out]
        n413 = call "Current Match Control.vi"("New Phase"=w557, "Mode"=T15."Set Phase") -> ()  [unwired: 8 in, 2 out]
      }
      event "Restore Session", "Continue Game Button": Value Change {
        n414 = event-data() -> ("CtlRef"=w565:refnum<vi>)  [unwired: 1 in]
        n415 = property class="Bool (strict)"(reference=w565, "Value"=FALSE) -> ()  [unwired: 1 in, 2 out]
        n416 = local read "Scoring Data File Path"() -> (w562:path)
        n417 = local read "Team Data File Path"() -> (w563:path)
        n418 = call <vilib>:"Check if File or Folder Exists.vi"("path"=w562) -> ("file or folder exists?"=w559:bool)  [unwired: 8 in, 2 out]
        n419 = call <vilib>:"Check if File or Folder Exists.vi"("path"=w563) -> ("file or folder exists?"=w560:bool)  [unwired: 8 in, 2 out]
        n420 = And(x=w560, y=w559) -> (x .and. y?=w561:bool)
        n421 = case shown="True" w561 {
          tunnel: w563 -> [_ w567]
          tunnel: w562 -> [_ w566]
          frame False {
            n422 = call "Display Message to User6"() -> ()  [unwired: 10 in, 2 out]
          }
          frame True {
            n423 = stacked-sequence {
              tunnel: w567 -> [w569 _]
              tunnel: w566 -> [w568 _]
              frame #0 {
                w572 = u16 2 items=["Get All", "Set", "Reset All", "Force Set", "Force Set All"] ("Get/Set Mode Selector")
                n424 = call-poly <vilib>:"Read From XML File.vi"("XML File Path"=w569) -> ("XML Elements"=w579:string)  [unwired: 8 in, 2 out]
                n425 = call-poly <vilib>:"Read From XML File.vi"("XML File Path"=w568) -> ("XML Elements"=w573:string)  [unwired: 8 in, 2 out]
                n426 = Unflatten From XML(xml string=w579, type=T6 [] ("Team Info")) -> (value=w576:T6)  [unwired: 1 in, 1 out]
                n427 = Unflatten From XML(xml string=w573, type=T9 [] ("Scores")) -> (value=w574:T9)  [unwired: 1 in, 1 out]
                n428 = call "ScoreControl.vi"("Get/Set Mode Selector"=w572) -> ("Scores"=w570:T9)  [unwired: 13 in, 1 out]
                n429 = call "Team Data Control.vi"("Mode"=T13."Clear All Teams") -> ("Team Array Out"=w577:T7[])  [unwired: 10 in]
                n430 = for {
                  tunnel: w577 -> [_]
                  tunnel: w576 -> [w582] mode=indexing
                  n431 = call "Team Data Control.vi"("Team Data To Add/Change"=w582, "Mode"=T13."Force Add Team") -> ()  [unwired: 9 in, 1 out]
                }
                n432 = flat-sequence {
                  tunnel: w574 -> [w581]
                  tunnel: w570 -> [_]
                  frame #0 {
                    w580 = u16 4 items=["Get All", "Set", "Reset All", "Force Set", "Force Set All"] ("Get/Set Mode Selector")
                    n433 = call "ScoreControl.vi"("Get/Set Mode Selector"=w580, "All Scores"=w581) -> ()  [unwired: 12 in, 2 out]
                  }
                }
              }
              frame #1 {
                w584 = T21."Enabled" ("Disabled")
                n434 = local write "Startup Navigation Tab Control"(enum32{"Start", "New", "Done", "Continue"}."Done" ("Startup Navigation Tab Control")) -> ()
                n435 = property on="System Monitor Button" class="Bool (strict)"("DisabledEnum"=w584) -> ()  [unwired: 2 in, 2 out]
                n436 = property on="View Rankings Button" class="Bool (strict)"("DisabledEnum"=w584) -> ()  [unwired: 2 in, 2 out]
                n437 = property on="Launch Score Entry" class="Bool (strict)"("DisabledEnum"=w584) -> ()  [unwired: 2 in, 2 out]
                n438 = property on="Go to Timekeeper Button" class="Bool (strict)"("DisabledEnum"=w584) -> ()  [unwired: 2 in, 2 out]
                n439 = property on="Settings Button" class="Bool (strict)"("DisabledEnum"=w584) -> ()  [unwired: 2 in, 2 out]
                n440 = property on="Profile Button" class="Bool (strict)"("DisabledEnum"=w584) -> ()  [unwired: 2 in, 2 out]
                n441 = property on="Local Entry Button" class="Bool (strict)"("DisabledEnum"=w584) -> ()  [unwired: 2 in, 2 out]
              }
            }
          }
        }
      }
      event "Local Entry Button": Value Change {
        n442 = event-data() -> ("CtlRef"=w587:refnum<vi>, "OldVal"=w586:bool)  [unwired: 1 in, 4 out]
        n443 = property class="Bool (strict)"(reference=w587, "Value"=w586) -> ()  [unwired: 1 in, 2 out]
        n444 = stacked-sequence {
          frame #0 {
            n445 = call "Team Data Control.vi"("Mode"=T13."Get Teams") -> ("Team Array Out"=w589:T7[])  [unwired: 10 in]
            n446 = for {
              tunnel: w589 -> [w592] mode=indexing
              tunnel: [w591] -> w588 mode=indexing
              n447 = Unbundle By Name(w592) -> ("Both"=w591:string)
            }
            n448 = property on="Select a Team for Manual Score Entry" class="Ring (strict)"("Strings []"=w588) -> ()  [unwired: 2 in, 2 out]
          }
          frame #1 {
            n449 = local read "Select a Team for Manual Score Entry"() -> (w594:u16)
            n450 = property on="Select a Team for Manual Score Entry" class="Ring (strict)"() -> ("Strings []"=w593:string[])  [unwired: 2 in, 2 out]
            n451 = Index Array(array=w593, index=w594) -> (element=w596:string)
            n452 = Decimal String To Number(string=w596) -> (number=w595:i32)  [unwired: 2 in, 1 out]
            n453 = call "Get_Next_Round.vi"("TeamNo"=w595) -> ("NextRound"=w597:u16)  [unwired: 10 in]
            n454 = Decrement(x=w597) -> (x-1=w598:u16)
            n455 = local write "ROUND"(w598) -> ()
          }
          frame #2 {
            n456 = local write "Splash Page Main Tab Control"(T12."Manual Score Entry" ("Splash Page Main Tab Control")) -> ()
            n457 = local write "Tab Control"(T5."Splash" ("Tab Control")) -> ()
          }
        }
      }
      event "Select a Team for Manual Score Entry": Value Change {
        n458 = event-data() -> ("NewVal"=w608:u16)  [unwired: 1 in, 5 out]
        n459 = property on="Select a Team for Manual Score Entry" class="Ring (strict)"() -> ("Strings []"=w609:string[])  [unwired: 2 in, 2 out]
        n460 = property on="SUBMIT Manual Score" class="Bool (strict)"("DisabledEnum"=T21."Enabled" ("Disabled")) -> ()  [unwired: 2 in, 2 out]
        n461 = Index Array(array=w609, index=w608) -> (element=w602:string)
        n462 = Decimal String To Number(string=w602) -> (number=w610:i32)  [unwired: 2 in, 1 out]
        n463 = call "Get_Next_Round.vi"("TeamNo"=w610) -> ("NextRound"=w601:u16)  [unwired: 10 in]
        n464 = Decrement(x=w601) -> (x-1=w603:u16)
        n465 = local write "ROUND"(w603) -> ()
        n466 = call "Find By Both.vi"("Both"=w602) -> ("Found?"=w604:bool, "Team Data"=w605:T7)  [unwired: 9 in]
        n467 = case shown="True" w604 {
          tunnel: w601 -> [_ w619]
          tunnel: w605 -> [_ w620]
          tunnel: [0 w616] -> w606
          frame False {
          }
          frame True {
            w621 = u16 0 items=["Automatic", "Manual"] ("Score Mode Selector")
            w622 = u16 0 items=["Get All", "Set", "Reset All", "Force Set", "Force Set All"] ("Get/Set Mode Selector")
            n468 = Unbundle By Name(w620) -> ("GUID"=w615:u16)
            n469 = call "ScoreControl.vi"("Get/Set Mode Selector"=w622, "GUID"=w615, "Round Number"=w619, "Score Mode Selector"=w621) -> ("Scores"=w614:T9)  [unwired: 10 in, 1 out]
            n470 = Array Size(array=w614) -> (size(s)=w613:i32)
            n471 = Greater Than 0?(x=w613) -> (x > 0?=w612:bool)
            n472 = case shown="True" w612 {
              tunnel: w619 -> [_ w629]
              tunnel: [FALSE w628] -> w618
              tunnel: [0.0 ("Score") w627] -> w617
              tunnel: w615 -> [_ w626]
              tunnel: w614 -> [_ w625]
              frame False {
              }
              frame True {
                n473 = for {
                  tunnel: w625 -> [w638] mode=indexing
                  tunnel: w629 -> [w636]
                  tunnel: [w630] -> w628
                  tunnel: [w635] -> w627
                  tunnel: w626 -> [w633]
                  stop <- w630 stop-if-true
                  n474 = Unbundle By Name(w638) -> ("Score.GUID"=w634:u16, "Score.Round Number"=w637:u16, "Score.Full Score Entry.Score"=w635:dbl)
                  n475 = Equal?(x=w637, y=w636) -> (x = y?=w632:bool)
                  n476 = Equal?(x=w634, y=w633) -> (x = y?=w631:bool)
                  n477 = And(x=w631, y=w632) -> (x .and. y?=w630:bool)
                }
              }
            }
            n478 = case shown="False" w618 {
              tunnel: w617 -> [_ w640]
              tunnel: [0 w640] -> w616
              frame False {
              }
              frame True {
              }
            }
          }
        }
        n479 = local write "Manual Score"(w606) -> ()
      }
      event "stop": Value Change {
        w641 = TRUE ("NewVal")
        n480 = event-data() -> ()  [unwired: 1 in, 3 out]
        n481 = local write "stop"(w641) -> ()
      }
      event "ROUND": Value Change {
        n482 = event-data() -> ("NewVal"=w649:u16)  [unwired: 1 in, 5 out]
        n483 = local read "Select a Team for Manual Score Entry"() -> (w647:u16)
        n484 = property on="Select a Team for Manual Score Entry" class="Ring (strict)"() -> ("Strings []"=w646:string[])  [unwired: 2 in, 2 out]
        n485 = Increment(x=w649) -> (x+1=w648:u16)
        n486 = Index Array(array=w646, index=w647) -> (element=w645:string)
        n487 = call "Find By Both.vi"("Both"=w645) -> ("Found?"=w644:bool, "Team Data"=w643:T7)  [unwired: 9 in]
        n488 = case shown="True" w644 {
          tunnel: w648 -> [_ w655]
          tunnel: w643 -> [_ w657]
          tunnel: [0 w652] -> w642
          frame False {
          }
          frame True {
            w658 = u16 0 items=["Automatic", "Manual"] ("Score Mode Selector")
            w659 = u16 0 items=["Get All", "Set", "Reset All", "Force Set", "Force Set All"] ("Get/Set Mode Selector")
            n489 = Unbundle By Name(w657) -> ("GUID"=w651:u16)
            n490 = call "ScoreControl.vi"("Get/Set Mode Selector"=w659, "GUID"=w651, "Round Number"=w655, "Score Mode Selector"=w658) -> ("Scores"=w656:T9)  [unwired: 10 in, 1 out]
            n491 = for {
              tunnel: w656 -> [w670] mode=indexing
              tunnel: w655 -> [w668]
              tunnel: [w664] -> w654
              tunnel: [w667] -> w653
              tunnel: w651 -> [w665]
              stop <- w662 stop-if-true
              n492 = Unbundle By Name(w670) -> ("Score.GUID"=w666:u16, "Score.Round Number"=w669:u16, "Score.Full Score Entry.Score"=w667:dbl)
              n493 = Equal?(x=w669, y=w668) -> (x = y?=w664:bool)
              n494 = Equal?(x=w666, y=w665) -> (x = y?=w663:bool)
              n495 = And(x=w663, y=w664) -> (x .and. y?=w662:bool)
            }
            n496 = case shown="False" w654 {
              tunnel: w653 -> [_ w661]
              tunnel: [0 w661] -> w652
              frame False {
              }
              frame True {
              }
            }
          }
        }
        n497 = local write "Manual Score"(w642) -> ()
      }
      event "SUBMIT Manual Score": Value Change {
        n498 = event-data() -> ("CtlRef"=w674:refnum<vi>, "OldVal"=w673:bool)  [unwired: 1 in, 4 out]
        n499 = local read "Select a Team for Manual Score Entry"() -> (w679:u16)
        n500 = property on="Select a Team for Manual Score Entry" class="Ring (strict)"() -> ("Strings []"=w678:string[])  [unwired: 2 in, 2 out]
        n501 = property class="Bool (strict)"(reference=w674, "Value"=w673) -> ()  [unwired: 1 in, 2 out]
        n502 = local read "ROUND"() -> (w672:u16)
        n503 = Index Array(array=w678, index=w679) -> (element=w677:string)
        n504 = Increment(x=w672) -> (x+1=w671:u16)
        n505 = call "Find By Both.vi"("Both"=w677) -> ("Found?"=w676:bool, "Team Data"=w675:T7)  [unwired: 9 in]
        n506 = case shown="True" w676 {
          tunnel: w671 -> [_ w680]
          tunnel: w675 -> [_ w681]
          frame False {
          }
          frame True {
            n507 = stacked-sequence {
              tunnel: w681 -> [w687 _]
              tunnel: w680 -> [w685 _]
              frame #0 {
                w688 = u16 1 items=["Automatic", "Manual"] ("Score Mode Selector")
                w689 = u16 3 items=["Get All", "Set", "Reset All", "Force Set", "Force Set All"] ("Get/Set Mode Selector")
                n508 = Unbundle By Name(w687) -> ("GUID"=w686:u16)
                n509 = local read "Manual Score"() -> (w683:dbl)
                n510 = Bundle By Name(cluster=T11 {"Elements"=[{"Name"="CO2 Balls Touching/Within Reservoir Model", "Value"="-1"}, {"Name"="Money Ball Touching/Within Reservoir Model", "Value"="-1"}, {"Name"="3+ Red/White Citizens in Pink Grid Area", "Value"="-1"}, {"Name"="# Upright Levee Blocks touching ONLY GREEN shores", "Value"="-1"}, {"Name"="# Upright Levee Blocks Touching any RED shore", "Value"="-1"}, {"Name"="Levee Test was Performed", "Value"="-1"}, {"Name"="Levee Test Wheel Blocked by NonLevee", "Value"="-1"}, {"Name"="Flood Barrier in Up Position", "Value"="-1"}, {"Name"="Both Yellow Arrows Aligned", "Value"="-1"}, {"Name"="Team Robot Touching Only Yellow Grid Area", "Value"="-1"}, {"Name"="Both Insulation Touching Green Grid Area", "Value"="-1"}, {"Name"="Bicycle Touching Green Grid Area", "Value"="-1"}, {"Name"="Computer Touching Green Grid Area", "Value"="-1"}, {"Name"="House in Up Position", "Value"="-1"}, {"Name"="House Window Showing Black", "Value"="-1"}, {"Name"="House Window All The Way Open", "Value"="-1"}, {"Name"="3+ Black/White Scientists Touching Research Area", "Value"="-1"}, {"Name"="Money Ball Touching/Within Research Area Model", "Value"="-1"}, {"Name"="Polar Bear Touching/Within Research Area Model", "Value"="-1"}, {"Name"="Polar Bear Orientation (Sleeping/Upright)", "Value"="-1"}, {"Name"="Ice Core Pulled From Its Hole", "Value"="-1"}, {"Name"="Ice Buoy Upright and Within/Touching Research Area Model", "Value"="-1"}, {"Name"="Drilling Machine Touching/Within Research Area Model", "Value"="-1"}, {"Name"="Drill Assembly Completely Vertical", "Value"="-1"}, {"Name"="Team Robot Touching/Within Research Area Model", "Value"="-1"}, {"Name"="3+ Blue/Gray Leaders Touching Green Mountain/City Area", "Value"="-1"}, {"Name"="Ice Core in Base Area", "Value"="-1"}, {"Name"="Snowmobile Touching/Within Research Area Model", "Value"="-1"}], "Score"=0.0} ("Full Score Entry"), "Score"=w683) -> (w682:T11)
                n511 = call "ScoreControl.vi"("Get/Set Mode Selector"=w689, "Full Score Entry"=w682, "GUID"=w686, "Round Number"=w685, "Score Mode Selector"=w688) -> ()  [unwired: 9 in, 2 out]
              }
              frame #1 {
                n512 = property on="SUBMIT Manual Score" class="Bool (strict)"("DisabledEnum"=T21."Disabled and Grayed Out" ("Disabled")) -> ()  [unwired: 2 in, 2 out]
              }
            }
          }
        }
      }
    }
  }
  n513 = while {
    tunnel: w6 -> [_]
    tunnel: w7 -> [w691]
    stop <- w692 stop-if-true
    n514 = stacked-sequence {
      tunnel: w691 -> [w693 _]
      frame #0 {
        n515 = Wait on Occurrence(2:w693) -> ()  [unwired: 2 in, 1 out]
      }
      frame #1 {
        n516 = call "File Dialog"("start path"="Scoring Data File Path", "prompt"="Write Human-Readable CSV File to:", "button label"="Save File", "pattern (all files)"="*.csv" ("pattern label"), "pattern label"="CSV Human Readable") -> ("selected path"=w701:path, "cancelled"=w700:bool, "error out"=w694:errorcluster)  [unwired: 7 in, 1 out]
        n517 = case shown="False" w700 {
          tunnel: w701 -> [w708 _]
          tunnel: "Rank,Team Number,Team Name,Highest Score,Match1,Match2,Match3,Match4 " -> [w705 _]
          tunnel: w694 -> [_ w733]
          frame False {
            n518 = Open/Create/Replace File(file path (use dialog)=w708, operation (0:open)=T26."replace or create with confirmation", access (0:read/write)=enum16{"read/write", "read-only", "write-only"}."write-only") -> (refnum out=w706:refnum<file>, error out=w707:errorcluster)  [unwired: 3 in, 1 out]
            n519 = case shown="No Error" w707 {
              tunnel: w707 -> [w713 _]
              tunnel: w706 -> [w714 _]
              tunnel: w705 -> [w711 _]
              frame No Error {
                n520 = property on="Team Rankings" class="Tbl (strict)"() -> ("Row Headers[]"=w722:string[])  [unwired: 2 in, 2 out]
                n521 = local read "Team Rankings"() -> (w721:string[][])
                n522 = for {
                  tunnel: w722 -> [w728] mode=indexing
                  tunnel: w721 -> [w725] mode=indexing
                  tunnel: "" -> [w726]
                  tunnel: [w723] -> w717 mode=indexing
                  n523 = for {
                    shift-right: [w729] -> w724
                    shift-left: w726 -> [w732]
                    tunnel: w725 -> [w730] mode=indexing
                    n524 = Concatenate Strings(w732, w730, "," ("string")) -> (w729:string)
                  }
                  n525 = Concatenate Strings(w728, "," ("string"), w724) -> (w723:string)
                }
                n526 = Concatenate Strings(w711, "\r\n") -> (w712:string)
                n527 = Write to Text File(file (use dialog)=w714, text=w712, error in=w713) -> (refnum out=w716:refnum<file>, error out=w715:errorcluster)  [unwired: 1 in, 1 out]
                n528 = Write to Text File(file (use dialog)=w716, text=w717, error in=w715) -> (refnum out=w718:refnum<file>, error out=w719:errorcluster)  [unwired: 1 in, 1 out]
                n529 = Close File(refnum=w718, error in=w719) -> (error out=w709:errorcluster)  [unwired: 1 out]
                n530 = case shown="Error" w709 {
                  frame No Error {
                    n531 = call "Display Message to User4"() -> ()  [unwired: 10 in, 2 out]
                  }
                  frame Error {
                    n532 = call "Display Message to User5"() -> ()  [unwired: 10 in, 2 out]
                  }
                }
              }
              frame Error {
                n533 = call "Display Message to User3"() -> ()  [unwired: 10 in, 2 out]
              }
            }
          }
          frame True {
            n534 = call <vilib>:"Clear Errors.vi"("error in (no error)"=w733) -> ()  [unwired: 6 in, 1 out]
          }
        }
      }
    }
    n535 = local read "stop"() -> (w692:bool)
  }
  n536 = call <vilib>:"OpenHandle.vi"() -> ("client handle out"=w12:T30, "error out"=w11:errorcluster)  [unwired: 14 in]
  n537 = while "Sound Handler Loop" {
    tunnel: w6 -> [_]
    stop <- w736 stop-if-true
    n538 = Wait (ms)(milliseconds to wait=u32 200) -> ()  [unwired: 1 out]
    n539 = local read "Sound Cluster"() -> (w739:T3)
    n540 = case shown="\"Hurry-Up\"" "Sound To Play" {
      tunnel: w739 -> [_ w778 w783 w788 w793 w798]
      tunnel: [T27 {"total number of samples/ch"=0, "sound format"={"sample rate (S/s)"=0.0, "number of channels"=0, "bits per sample"=0}, "data"=[], "Volume"=0.0} ("Uh-Oh") w777 w782 w786 w791 w796] -> w738
      tunnel: [FALSE TRUE TRUE TRUE TRUE TRUE] -> w737
      tunnel: [0.0 ("Pre-Match Coundown Sound Volume") w774 w779 w784 w789 w794] -> w734
      frame "None", Default {
      }
      frame "Start" {
        n541 = local read "Start Sound Volume"() -> (w774:dbl)
        n542 = local write "Sound To Play"(enum16{"None", "Start", "Stop", "Uh-Oh"}."None" ("Sound To Play")) -> ()
        n543 = Unbundle By Name(w778) -> ("Start"=w777:T27)
      }
      frame "Stop" {
        n544 = Unbundle By Name(w783) -> ("Stop"=w782:T27)
        n545 = local read "Stop Sound Volume"() -> (w779:dbl)
        n546 = local write "Sound To Play"(enum16{"None", "Start", "Stop", "Uh-Oh"}."None" ("Sound To Play")) -> ()
      }
      frame "Uh-Oh" {
        n547 = local write "Sound To Play"(enum16{"None", "Start", "Stop", "Uh-Oh"}."None" ("Sound To Play")) -> ()
        n548 = local read "Uh-Oh Sound Volume"() -> (w784:dbl)
        n549 = Unbundle By Name(w788) -> ("Uh-Oh"=w786:T27)
      }
      frame "Prematch" {
        n550 = local read "Pre-Match Coundown Sound Volume"() -> (w789:dbl)
        n551 = local write "Sound To Play"(enum16{"None", "Start", "Stop", "Uh-Oh"}."None" ("Sound To Play")) -> ()
        n552 = Unbundle By Name(w793) -> ("PreMatch"=w791:T27)
      }
      frame "Hurry-Up" {
        n553 = local read "Hurry-Up Sound Volume"() -> (w794:dbl)
        n554 = local write "Sound To Play"(enum16{"None", "Start", "Stop", "Uh-Oh"}."None" ("Sound To Play")) -> ()
        n555 = Unbundle By Name(w798) -> ("Hurry-Up"=w796:T27)
      }
    }
    n556 = case shown="True" w737 {
      tunnel: w738 -> [_ w761]
      tunnel: w734 -> [_ w741]
      frame False {
      }
      frame True {
        w759 = T31 0 items=["Finite Samples", "Continuous Samples"] ("sample mode")
        n557 = Unbundle By Name(w761) -> ("total number of samples/ch"=w760:u32, "sound format"=w758:T4, "data"=w751:waveform(dbl)[])
        n558 = Divide(x="Master Volume", y=100.0) -> (x/y=w744:dbl)
        n559 = Multiply(x=w741, y=w744) -> (x*y=w743:dbl)
        n560 = call <vilib>:"Sound Output Configure.vi"("number of samples/ch"=w760, "sample mode"=w759, "sound format"=w758, "device ID"=u32 0) -> ("error out"=w756:errorcluster, "task ID"=w757:T32)  [unwired: 6 in]
        n561 = call-poly <vilib>:"Sound Output Set Volume.vi"("error in (no error)"=w756, "volume"=w743, "task ID"=w757) -> ("error out"=w754:errorcluster, "task ID out"=w755:T32)  [unwired: 7 in]
        n562 = call <vilib>:"Sound Output Start.vi"("error in (no error)"=w754, "task ID"=w755) -> ("error out"=w752:errorcluster, "task ID out"=w753:T32)  [unwired: 8 in]
        n563 = call-poly <vilib>:"Sound Output Write.vi"("error in (no error)"=w752, "data"=w751, "task ID"=w753) -> ("error out"=w749:errorcluster, "task ID out"=w750:T32)  [unwired: 7 in]
        n564 = while {
          tunnel: w750 -> [w770]
          tunnel: w749 -> [w769]
          tunnel: [w768] -> w748
          tunnel: [w767] -> w747
          stop <- w762 continue-if-true
          n565 = call <vilib>:"Sound Output Info.vi"("error in (no error)"=w769, "task ID"=w770) -> ("error out"=w767:errorcluster, "is playing?"=w766:bool, "task ID out"=w768:T32)  [unwired: 6 in, 1 out]
          n566 = local read "Sound To Play"() -> (w764:T2)
          n567 = Equal?(x=w764, y=enum16{"None", "Start", "Stop", "Uh-Oh"}."None") -> (x = y?=w765:bool)
          n568 = And(x=w766, y=w765) -> (x .and. y?=w762:bool)
        }
        n569 = call <vilib>:"Sound Output Stop.vi"("error in (no error)"=w747, "task ID"=w748) -> ()  [unwired: 8 in, 2 out]
      }
    }
    n570 = local read "stop"() -> (w736:bool)
  }
  n571 = while "Timer Loop" {
    tunnel: w6 -> [_]
    stop <- w828 stop-if-true
    n572 = Wait (ms)(milliseconds to wait=u32 100) -> ()  [unwired: 1 out]
    n573 = Bundle By Name(cluster=T33 {"Primary"=0.0, "Secondary"=0.0, "Pre-Primary"=0.0} ("Time Settings"), "Primary"="Primary (s)", "Secondary"="Secondary (s)", "Pre-Primary"="Pre-Primary (s)") -> (w830:T33)
    n574 = Build Array("Primary (s)", 0.0 ("element"), 30.0 ("element")) -> (w823:dbl[])
    n575 = Build Array("Pre-Primary (s)") -> (w811:dbl[])
    n576 = call "Timer Running Control.vi"("Enum"=T14."Get Timer State") -> ("Timer State"=w817:bool)  [unwired: 10 in]
    n577 = call "Timer.vi"("PreMatchMetThisCycle?"=w811, "PrimaryMetThisCycle?"=w823, "Time Settings"=w830, "Run?"=w817) -> ("Stopped"=w813:bool, "Time Remaining"=w799:dbl, "Unexpected Reset"=w826:bool, "PrimaryMetThisCycle"=w804:bool[], "PreMatchMetThisCycle"=w809:bool[], "State"=w815:T16)  [unwired: 2 in]
    n578 = Index Array(array=w809, index=0) -> (element=w801:bool)
    n579 = Greater Than 0?(x=w799) -> (x > 0?=w800:bool)
    n580 = And(x=w801, y=w800) -> (x .and. y?=w802:bool)
    n581 = case shown="True" w802 {
      frame False {
      }
      frame True {
        w835 = T35."Prematch" ("Sound To Play")
        n582 = call "GetSetProfileInfo.vi"("Parameter"=T34."LastSound", "Get/Set State"=enum16{"Get", "Set", "Load"}."Set", "LastSoundIn"=w835) -> ()  [unwired: 4 in, 5 out]
        n583 = local write "Sound To Play"(w835) -> ()
      }
    }
    n584 = case shown="\"Secondary\"" w815 {
      tunnel: [u32 16711680 u32 6618880 u32 16711680 u32 16774656] -> w808
      frame "Stopped", Default {
      }
      frame "Primary" {
      }
      frame "Secondary" {
      }
      frame "Pre-Primary" {
      }
    }
    n585 = case shown="True" w826 {
      frame False {
      }
      frame True {
        w846 = enum16{"None", "Start", "Stop", "Uh-Oh"}."Uh-Oh" ("Sound To Play")
        n586 = call "GetSetProfileInfo.vi"("Parameter"=T34."LastSound", "Get/Set State"=enum16{"Get", "Set", "Load"}."Set", "LastSoundIn"=w846) -> ()  [unwired: 4 in, 5 out]
        n587 = local write "Sound To Play"(w846) -> ()
      }
    }
    n588 = Index Array(array=w804, index=0) -> (element=w821:bool)
    n589 = Index Array(array=w804, index=1) -> (element=w819:bool)
    n590 = Index Array(array=w804, index=2) -> (element=w806:bool)
    n591 = call "State Control.vi"("State"=w815, "Action"=enum16{"Get", "Set"}."Set") -> ()  [unwired: 9 in, 1 out]
    n592 = case shown="True" w821 {
      frame False {
      }
      frame True {
        w845 = enum16{"None", "Start", "Stop", "Uh-Oh"}."Start" ("Sound To Play")
        n593 = call "GetSetProfileInfo.vi"("Parameter"=T34."LastSound", "Get/Set State"=enum16{"Get", "Set", "Load"}."Set", "LastSoundIn"=w845) -> ()  [unwired: 4 in, 5 out]
        n594 = local write "Sound To Play"(w845) -> ()
      }
    }
    n595 = case shown="True" w819 {
      frame False {
      }
      frame True {
        w840 = enum16{"None", "Start", "Stop", "Uh-Oh"}."Stop" ("Sound To Play")
        n596 = call "GetSetProfileInfo.vi"("Parameter"=T34."LastSound", "Get/Set State"=enum16{"Get", "Set", "Load"}."Set", "LastSoundIn"=w840) -> ()  [unwired: 4 in, 5 out]
        n597 = local write "Sound To Play"(w840) -> ()
      }
    }
    n598 = case shown="True" w806 {
      frame False {
      }
      frame True {
        w832 = T2."Hurry-Up" ("Sound To Play")
        n599 = call "GetSetProfileInfo.vi"("Parameter"=T34."LastSound", "Get/Set State"=enum16{"Get", "Set", "Load"}."Set", "LastSoundIn"=w832) -> ()  [unwired: 4 in, 5 out]
        n600 = local write "Sound To Play"(w832) -> ()
      }
    }
    n601 = case shown="True" w813 {
      frame False {
      }
      frame True {
        n602 = call "Current Match Control.vi"("Mode"=T15."Increment") -> ("Current Match"=→"Current Match":u16)  [unwired: 9 in, 1 out]
      }
    }
    n603 = property on="Time Remaining" class="Str"("Text.BGColor"=w808) -> ()  [unwired: 2 in, 2 out]
    n604 = local read "stop"() -> (w828:bool)
    n605 = call "Number to Time String.vi"("Numeric"=w799) -> ("String"=→"Time Remaining":string)  [unwired: 10 in]
    n606 = call "Time Remaining Control.vi"("Numeric"=w799, "Mode"=enum16{"Get", "Set"}."Set") -> ()  [unwired: 9 in, 1 out]
  }
  n607 = flat-sequence "Queue Checkers" {
    tunnel: w6 -> [_]
    frame #0 {
      w855 = string[][] []  # Score Log
      w856 = string[][] []  # Timer Log
      w873 = string[][] []  # Error Log
      n608 = Obtain Queue(name (unnamed)="Score File Queue", element data type=T36 {"Scoring Data"=[], "Round"=0, "GUID"=0, "GUSID"="", "Time Stamp"=timestamp(0 s since 1904-01-01), "Submitter"=""} ("Cluster")) -> (queue out=w861:refnum<queue>, error out=w860:errorcluster)  [unwired: 3 in, 1 out]
      n609 = Obtain Queue(name (unnamed)="Error File Queue", element data type=T37 {"Filename"="", "File Contents"="", "Time Stamp"=timestamp(0 s since 1904-01-01), "Origin"=""} ("Cluster")) -> (queue out=w865:refnum<queue>, error out=w866:errorcluster)  [unwired: 3 in, 1 out]
      n610 = Obtain Queue(name (unnamed)="Log Queue", element data type=T38 {"Time Stamp"=timestamp(0 s since 1904-01-01), "Origin"="", "Message"="", "Log"=enum."Error Log"} ("Cluster")) -> (queue out=w870:refnum<queue>, error out=w869:errorcluster)  [unwired: 3 in, 1 out]
      n611 = while "Score File Handler" {
        tunnel: w861 -> [w887]
        tunnel: w860 -> [w886]
        tunnel: [w881] -> w859
        tunnel: [w880] -> w858
        stop <- w884 stop-if-true
        n612 = Dequeue Element(queue=w887, timeout in ms (-1)=100, error in (no error)=w886) -> (queue out=w875:refnum<queue>, element=w882:T36, timed out?=w883:bool, error out=w880:errorcluster)
        n613 = Get Queue Status(queue=w875, return elements? (F)=FALSE) -> (queue out=w874:refnum<queue>, max queue size=w876:i32, # elements in queue=w877:i32)  [unwired: 1 in, 5 out]
        n614 = Equal?(x=w876, y=w877) -> ()  [unwired: 1 out]
        n615 = case shown="False" w883 {
          tunnel: w882 -> [w919 _]
          tunnel: w874 -> [w920 w930]
          tunnel: [w920 w930] -> w881
          tunnel: "Score Folder" -> [w912 _]
          frame False {
            n616 = Unbundle By Name(w919) -> ("GUSID"=w888:string, "Time Stamp"=w908:timestamp, "Submitter"=w904:string, "GUID"=w902:u16, "Round"=w900:u16, "Scoring Data"=w898:cluster{"Name":string, "Value":string}[])
            n617 = Number To Decimal String(number=w902) -> (decimal integer string=w895:string)  [unwired: 1 in]
            n618 = Number To Decimal String(number=w900) -> (decimal integer string=w893:string)  [unwired: 1 in]
            n619 = for {
              tunnel: w898 -> [w929] mode=indexing
              shift-right: [w922] -> w896
              shift-left: "" -> [w923]
              n620 = Unbundle By Name(w929) -> ("Name"=w927:string, "Value"=w925:string)
              n621 = Concatenate Strings(w923, "\"" ("string"), w927, "\":\"" ("string"), w925, "\"" ("string"), "\r\n") -> (w922:string)
            }
            n622 = Concatenate Strings(w895, "." ("string"), w893, "." ("string"), w888) -> (w890:string)
            n623 = Format Date/Time String(time format string (%c)="%y.%m.%d %H:%M:%S", seconds (now)=w908) -> (date/time string=w907:string)  [unwired: 1 in]
            n624 = Concatenate Strings(w890, ".txt" ("string")) -> (w910:string)
            n625 = Build Path(base path=w912, name or relative path=w910) -> (appended path=w909:path)
            n626 = Concatenate Strings("At " ("string"), w907, ", " ("string"), w904, " submitted the following for GUID " ("string"), w895, ", round " ("string"), w893, ":" ("string"), "\r\n", w896) -> (w891:string)
            n627 = Open/Create/Replace File(file path (use dialog)=w909, operation (0:open)=T26."create") -> (refnum out=w917:refnum<file>, error out=w916:errorcluster)  [unwired: 4 in, 1 out]
            n628 = Write to Text File(file (use dialog)=w917, text=w891, error in=w916) -> (refnum out=w915:refnum<file>, error out=w914:errorcluster)  [unwired: 1 in, 1 out]
            n629 = Close File(refnum=w915, error in=w914) -> ()  [unwired: 2 out]
          }
          frame True {
          }
        }
        n630 = local read "stop"() -> (w884:bool)
      }
      n631 = while "Error File Handler" {
        tunnel: w865 -> [w945]
        tunnel: w866 -> [w944]
        tunnel: [w939] -> w867
        tunnel: [w937] -> w868
        stop <- w942 stop-if-true
        n632 = Dequeue Element(queue=w945, timeout in ms (-1)=100, error in (no error)=w944) -> (queue out=w933:refnum<queue>, element=w940:T37, timed out?=w941:bool, error out=w937:errorcluster)
        n633 = Get Queue Status(queue=w933, return elements? (F)=FALSE) -> (queue out=w932:refnum<queue>, max queue size=w934:i32, # elements in queue=w935:i32)  [unwired: 1 in, 5 out]
        n634 = Equal?(x=w934, y=w935) -> (x = y?=→"Error Queue Full":bool)
        n635 = case shown="False" w941 {
          tunnel: w940 -> [w965 _]
          tunnel: w932 -> [w966 w983]
          tunnel: [w966 w983] -> w939
          tunnel: "Error Folder" -> [w948 _]
          frame False {
            n636 = Unbundle By Name(w965) -> ("Filename"=w949:string, "File Contents"=w956:string, "Time Stamp"=w964:timestamp, "Origin"=w959:string)
            n637 = while {
              tunnel: w948 -> [w976]
              tunnel: w949 -> [w973]
              shift-right: [w969] -> _
              shift-left: "" -> [w971]
              tunnel: [w968] -> w946
              i -> [w970]
              stop <- w977 continue-if-true
              n638 = Concatenate Strings(w973, w971, ".txt" ("string")) -> (w974:string)
              n639 = Build Path(base path=w976, name or relative path=w974) -> (appended path=w972:path)
              n640 = call <vilib>:"Check if File or Folder Exists.vi"("path"=w972) -> ("file or folder exists?"=w977:bool, "dup path"=w967:path)  [unwired: 8 in, 1 out]
              n641 = case shown="True" w977 {
                tunnel: w970 -> [_ w982]
                tunnel: ["" w981] -> w969
                tunnel: [w978 w980] -> w968
                tunnel: w967 -> [w978 w980]
                frame False {
                }
                frame True {
                  n642 = Number To Decimal String(number=w982) -> (decimal integer string=w981:string)  [unwired: 1 in]
                }
              }
            }
            n643 = Format Date/Time String(time format string (%c)="%y.%m.%d %H:%M:%S", seconds (now)=w964) -> (date/time string=w961:string)  [unwired: 1 in]
            n644 = Concatenate Strings("At " ("string"), w961, ", " ("string"), w959, " wrote:" ("string"), "\r\n", w956) -> (w955:string)
            n645 = Open/Create/Replace File(file path (use dialog)=w946, operation (0:open)=T26."create") -> (refnum out=w954:refnum<file>, error out=w953:errorcluster)  [unwired: 4 in, 1 out]
            n646 = Write to Text File(file (use dialog)=w954, text=w955, error in=w953) -> (refnum out=w952:refnum<file>, error out=w951:errorcluster)  [unwired: 1 in, 1 out]
            n647 = Close File(refnum=w952, error in=w951) -> ()  [unwired: 2 out]
          }
          frame True {
          }
        }
        n648 = local read "stop"() -> (w942:bool)
      }
      n649 = while "Logging Loop" {
        tunnel: w870 -> [w1018]
        tunnel: [w994] -> w854
        shift-right: [w992] -> w853
        shift-left: w869 -> [w1017]
        shift-right: [w1001] -> _
        shift-left: w873 -> [w1002]
        shift-right: [w998] -> _
        shift-left: w856 -> [w999]
        shift-right: [w996] -> _
        shift-left: w855 -> [w997]
        stop <- w1019 stop-if-true
        n650 = Dequeue Element(queue=w1018, timeout in ms (-1)=100, error in (no error)=w1017) -> (queue out=w995:refnum<queue>, element=w1016:T38, timed out?=w1004:bool, error out=w993:errorcluster)
        n651 = Unbundle By Name(w1016) -> ("Log"=w1000:enum16{"Error Log", "Timer Log", "Scoring Log"}, "Time Stamp"=w1012:timestamp, "Origin"=w1008:string, "Message"=w1006:string)
        n652 = Format Date/Time String(time format string (%c)="%y.%m.%d %H:%M:%S", seconds (now)=w1012) -> (date/time string=w1010:string)  [unwired: 1 in]
        n653 = Format Date/Time String(time format string (%c)="%H:%M:%S", seconds (now)=w1012) -> (date/time string=w1014:string)  [unwired: 1 in]
        n654 = Build Array(w1014, w1008, w1006) -> (w1003:string[])
        n655 = call <vilib>:"Space Constant.vi"() -> ("String"=w1009:string)
        n656 = Concatenate Strings(w1010, w1009, w1008, "::" ("string"), w1006, "\r\n") -> (w1005:string)
        n657 = case shown="False" w1004 {
          tunnel: w1005 -> [w1031 _]
          tunnel: w1003 -> [w1030 _]
          tunnel: w1002 -> [w1029 w1097]
          tunnel: [w1028 w1097] -> w1001
          tunnel: w1000 -> [w1027 _]
          tunnel: "Error Logfile Path" -> [w1026 _]
          tunnel: "Timing Logfile Path" -> [w1025 _]
          tunnel: w999 -> [w1024 w1096]
          tunnel: [w1023 w1096] -> w998
          tunnel: w997 -> [w1022 w1095]
          tunnel: [w1021 w1095] -> w996
          tunnel: "Scoring Logfile Path" -> [w1020 _]
          frame False {
            n658 = case shown="\"Error Log\", Default" w1027 {
              tunnel: w1031 -> [w1042 w1062 w1078]
              tunnel: w1030 -> [w1041 w1059 w1080]
              tunnel: w1029 -> [w1040 w1061 w1081]
              tunnel: [w1035 w1061 w1081] -> w1028
              tunnel: w1026 -> [w1036 _ _]
              tunnel: w1025 -> [_ w1060 _]
              tunnel: w1024 -> [w1034 w1058 w1082]
              tunnel: [w1034 w1056 w1082] -> w1023
              tunnel: w1022 -> [w1033 w1057 w1079]
              tunnel: [w1033 w1057 w1076] -> w1021
              tunnel: w1020 -> [_ _ w1077]
              frame "Error Log", Default {
                n659 = Build Array (concatenate)(w1041, w1040) -> (w1035:string[][])
                "Error Log" <- w1035
                n660 = Open/Create/Replace File(file path (use dialog)=w1036, operation (0:open)=T26."open or create", access (0:read/write)=enum16{"read/write", "read-only", "write-only"}."write-only") -> (refnum out=w1038:refnum<file>, error out=w1037:errorcluster)  [unwired: 3 in, 1 out]
                n661 = case shown="No Error" w1037 {
                  selector: w1037 -> [w1046 _]
                  tunnel: w1042 -> [w1047 _]
                  tunnel: w1038 -> [w1045 _]
                  frame No Error {
                    n662 = Get File Size(file=w1045, error in=w1046) -> (refnum out=w1052:refnum<file>, size (in bytes)=w1050:i64, 0:w1051:errorcluster)
                    n663 = Set File Position(offset (in bytes) (0)=w1050, refnum=w1052, error in=w1051) -> (refnum out=w1049:refnum<file>, error out=w1048:errorcluster)  [unwired: 1 in]
                    n664 = Write to Text File(file (use dialog)=w1049, text=w1047, error in=w1048) -> (refnum out=w1044:refnum<file>, error out=w1043:errorcluster)  [unwired: 1 in, 1 out]
                    n665 = Close File(refnum=w1044, error in=w1043) -> ()  [unwired: 2 out]
                  }
                  frame Error {
                  }
                }
              }
              frame "Timer Log" {
                n666 = Build Array (concatenate)(w1059, w1058) -> (w1056:string[][])
                "Timer Log" <- w1056
                n667 = Open/Create/Replace File(file path (use dialog)=w1060, operation (0:open)=T26."open or create", access (0:read/write)=enum16{"read/write", "read-only", "write-only"}."write-only") -> (refnum out=w1055:refnum<file>, error out=w1054:errorcluster)  [unwired: 3 in, 1 out]
                n668 = case shown="No Error" w1054 {
                  selector: w1054 -> [w1064 _]
                  tunnel: w1062 -> [w1066 _]
                  tunnel: w1055 -> [w1065 _]
                  frame No Error {
                    n669 = Get File Size(file=w1065, error in=w1064) -> (refnum out=w1073:refnum<file>, size (in bytes)=w1071:i64, 0:w1072:errorcluster)
                    n670 = Set File Position(offset (in bytes) (0)=w1071, refnum=w1073, error in=w1072) -> (refnum out=w1070:refnum<file>, error out=w1069:errorcluster)  [unwired: 1 in]
                    n671 = Write to Text File(file (use dialog)=w1070, text=w1066, error in=w1069) -> (refnum out=w1068:refnum<file>, error out=w1067:errorcluster)  [unwired: 1 in, 1 out]
                    n672 = Close File(refnum=w1068, error in=w1067) -> ()  [unwired: 2 out]
                  }
                  frame Error {
                  }
                }
              }
              frame "Scoring Log" {
                n673 = Build Array (concatenate)(w1080, w1079) -> (w1076:string[][])
                "Scoring Log" <- w1076
                n674 = Open/Create/Replace File(file path (use dialog)=w1077, operation (0:open)=T26."open or create", access (0:read/write)=enum16{"read/write", "read-only", "write-only"}."write-only") -> (refnum out=w1083:refnum<file>, error out=w1075:errorcluster)  [unwired: 3 in, 1 out]
                n675 = case shown="No Error" w1075 {
                  selector: w1075 -> [w1085 _]
                  tunnel: w1083 -> [w1087 _]
                  tunnel: w1078 -> [w1086 _]
                  frame No Error {
                    n676 = Get File Size(file=w1087, error in=w1085) -> (refnum out=w1094:refnum<file>, size (in bytes)=w1092:i64, 0:w1093:errorcluster)
                    n677 = Set File Position(offset (in bytes) (0)=w1092, refnum=w1094, error in=w1093) -> (refnum out=w1091:refnum<file>, error out=w1090:errorcluster)  [unwired: 1 in]
                    n678 = Write to Text File(file (use dialog)=w1091, text=w1086, error in=w1090) -> (refnum out=w1089:refnum<file>, error out=w1088:errorcluster)  [unwired: 1 in, 1 out]
                    n679 = Close File(refnum=w1089, error in=w1088) -> ()  [unwired: 2 out]
                  }
                  frame Error {
                  }
                }
              }
            }
          }
          frame True {
          }
        }
        n680 = Get Queue Status(queue=w995, return elements? (F)=FALSE, error in (no error)=w993) -> (queue out=w994:refnum<queue>, max queue size=w989:i32, error out=w992:errorcluster, # elements in queue=w990:i32)  [unwired: 4 out]
        n681 = Equal?(x=w989, y=w990) -> (x = y?=→"Log Queue Full":bool)
        n682 = local read "stop"() -> (w1019:bool)
      }
      n683 = Release Queue(queue=w859, error in (no error)=w858) -> ()  [unwired: 1 in, 3 out]
      n684 = Release Queue(queue=w867, error in (no error)=w868) -> ()  [unwired: 1 in, 3 out]
      n685 = Release Queue(queue=w854, error in (no error)=w853) -> ()  [unwired: 1 in, 3 out]
    }
  }
  n686 = while "Check Network Stuff" {
    tunnel: w6 -> [_]
    tunnel: w12 -> [w1100]
    tunnel: w11 -> [w1099]
    tunnel: [w1098] -> w10
    tunnel: [w1101] -> w9
    i -> [w1104]
    stop <- w1106 stop-if-true
    n687 = Quotient & Remainder(x=w1104, y=2) -> (x-y*floor(x/y)=w1102:i32)  [unwired: 1 out]
    n688 = Wait (ms)(milliseconds to wait=u32 1000) -> ()  [unwired: 1 out]
    n689 = case shown="0, Default" w1102 {
      tunnel: [w1111 w1128] -> w1101
      tunnel: w1100 -> [w1110 w1128]
      tunnel: w1099 -> [w1109 _]
      tunnel: [w1108 errorcluster {"status"=FALSE, "code"=0, "source"=""} ("error IO")] -> w1098
      frame 0, Default {
        n690 = local read "Port"() -> (w1107:string)
        n691 = Concatenate Strings("http://localhost:" ("string"), w1107, "/FLL/" ("string")) -> (w1115:string)
        n692 = call <vilib>:"GET.vi"("client handle"=w1110, "url"=w1115, "error in (no error)"=w1109) -> ("client handle out"=w1111:T30, "headers"=w1113:string, "error out"=w1116:errorcluster)  [unwired: 9 in, 1 out]
        n693 = case shown="No Error" w1116 {
          selector: w1116 -> [w1118 w1124]
          tunnel: [TRUE FALSE] -> w1112
          tunnel: w1113 -> [w1119 _]
          tunnel: [w1118 w1124] -> w1108
          frame No Error {
            n694 = Match Pattern(string=w1119, regular expression="404 Not Found") -> (offset past match=w1122:i32)  [unwired: 1 in, 3 out]
            n695 = Less Than 0?(x=w1122) -> (x < 0?=→"Web Pages Not Found":bool)
          }
          frame Error {
          }
        }
        "Server Running" <- w1112
      }
      frame 1 {
        n696 = String To IP() -> (0:w1126:u32[])  [unwired: 1 in]
        n697 = for {
          tunnel: w1126 -> [w1132] mode=indexing
          tunnel: [w1130] -> w1129
          stop <- w1136 stop-if-true
          n698 = IP To String(1:TRUE ("dot notation? (F)"), 2:w1132) -> (0:w1131:string)
          n699 = local read "Current IP"() -> (w1135:string)
          n700 = Not Equal?(x=w1135, y="127.0.0.1") -> (x != y?=w1130:bool)
          n701 = Equal?(x=w1135, y=w1131) -> (x = y?=w1136:bool)
        }
        "Network Interface Up" <- w1129
      }
    }
    n702 = local read "stop"() -> (w1106:bool)
  }
  n703 = while {
    tunnel: w14 -> [w1140]
    tunnel: w6 -> [_]
    shift-right: [w1137] -> _
    shift-left: u32[] [] -> [w1138]
    stop <- w1141 stop-if-true
    n704 = event shown="[1] <Is Changed>: User Event" {
      selector: w1140 -> [_ _ _]
      dyn-events: _ -> [_ _ _]
      timeout: 1000 -> [_ _ _]
      tunnel: w1138 -> [w1142 w1144 w1172]
      tunnel: [w1142 w1143 w1172] -> w1137
      event Timeout {
        n705 = event-data() -> ()  [unwired: 1 in, 2 out]
      }
      event User Event {
        n706 = event-data() -> ()  [unwired: 1 in, 4 out]
        n707 = flat-sequence {
          tunnel: [w1147] -> w1146
          tunnel: w1146 -> [w1149]
          tunnel: [w1149] -> w1145
          tunnel: w1145 -> [w1168]
          tunnel: w1144 -> [w1167]
          tunnel: [w1165] -> w1143
          frame #0 {
            n708 = Tick Count (ms)() -> (millisecond timer value=w1147:u32)
            "Write Scores to file indicator" <- TRUE ("Write Scores to file indicator")
          }
          frame #1 {
            n709 = local read "Scoring Data File Path"() -> (w1150:path)
            n710 = disable-structure shown="Enabled" {
              disable-tunnel: w1150 -> [w1151 w1158 w1162]
              frame Disabled {
                n711 = call "Write Score Data To File.vi"("XML File Path"=w1151) -> ()  [unwired: 10 in, 1 out]
              }
              frame Disabled {
                w1160 = u16 0 items=["Get All", "Set", "Reset All", "Force Set", "Force Set All"] ("Get/Set Mode Selector")
                n712 = call "ScoreControl.vi"("Get/Set Mode Selector"=w1160) -> ("Scores"=w1159:T9)  [unwired: 13 in, 1 out]
                n713 = Flatten To XML(anything=w1159) -> (xml string=w1154:string)
                n714 = Open/Create/Replace File(file path (use dialog)=w1158, operation (0:open)=T26."replace or create") -> (refnum out=w1156:refnum<file>, error out=w1155:errorcluster)  [unwired: 4 in, 1 out]
                n715 = Write to Text File(file (use dialog)=w1156, text=w1154, error in=w1155) -> (refnum out=w1153:refnum<file>, error out=w1152:errorcluster)  [unwired: 1 in, 1 out]
                n716 = Close File(refnum=w1153, error in=w1152) -> ()  [unwired: 2 out]
              }
              frame Enabled {
                w1164 = u16 0 items=["Get All", "Set", "Reset All", "Force Set", "Force Set All"] ("Get/Set Mode Selector")
                n717 = call "ScoreControl.vi"("Get/Set Mode Selector"=w1164) -> ("Scores"=w1163:T9)  [unwired: 13 in, 1 out]
                n718 = Flatten To XML(anything=w1163) -> (xml string=w1161:string)
                n719 = call-poly <vilib>:"Write to XML File.vi"("XML Input"=w1161, "XML File Path"=w1162) -> ()  [unwired: 7 in, 3 out]
              }
            }
          }
          frame #2 {
            n720 = local write "Write Scores to file indicator"(FALSE ("Write Scores to file indicator")) -> ()
            n721 = Tick Count (ms)() -> (millisecond timer value=w1169:u32)
            n722 = Subtract(x=w1169, y=w1168) -> (x-y=w1166:u32)
            n723 = Build Array (concatenate)(w1167, w1166) -> (w1165:u32[])
          }
        }
      }
      event "Boolean": Value Change {
        n724 = event-data() -> ()  [unwired: 1 in, 4 out]
        n725 = Array Max & Min(array=w1172) -> (max value=→"max value":u32, min value=→"min value":u32)  [unwired: 2 out]
        n726 = call-poly <vilib>:"Mean.vi"("X"=w1172) -> ("mean"=→"mean":dbl)  [unwired: 1 out]
      }
    }
    n727 = local read "stop"() -> (w1141:bool)
  }
  n728 = call <vilib>:"CloseHandle.vi"("client handle"=w9, "error in (no error)"=w10) -> ()  [unwired: 13 in, 1 out]
  n729 = while {
    tunnel: w2 -> [w1175]
    stop <- w1176 stop-if-true
    n730 = stacked-sequence {
      tunnel: w1175 -> [w1177 _]
      frame #0 {
        n731 = Wait on Occurrence(2:w1177) -> ()  [unwired: 2 in, 1 out]
      }
      frame #1 {
        w1183 = T40 {"Team Info"=[], "Match Array (indices)"=[]} ("TeamData_and_Schedule IN")
        n732 = Unbundle(w1183) -> ("Team Info"=w1180:T41)  [unwired: 1 out]
        n733 = Array To Cluster(array=w1180) -> (cluster=w1181:T42)
        n734 = Unbundle(w1181) -> ("Team Info[0]"=w1182:T43)
        n735 = call "Team Data Control.vi"("Mode"=T24."Get Teams") -> ("Team Array Out"=w1179:T7[])  [unwired: 10 in]
        n736 = for {
          tunnel: w1179 -> [w1223] mode=indexing
          tunnel: w1182 -> [w1222]
          tunnel: [w1217] -> w1184 mode=indexing
          n737 = Unbundle By Name(w1223) -> ("Both"=w1221:string, "Name"=w1220:string, "GUID"=w1219:u16, "Number"=w1218:u16)
          n738 = Bundle By Name(cluster=w1222, "Both"=w1221, "Name"=w1220, "GUID"=w1219, "Number"=w1218) -> (w1217:T43)
        }
        n739 = local read "Scores Exist"() -> (w1188:bool)
        n740 = Not(x=w1188) -> (.not. x?=w1189:bool)
        n741 = Bundle(cluster=w1183, "Team Info"=w1184) -> (w1185:T40)  [unwired: 1 in]
        n742 = call "Team Editor and Schedule Creator.vi"("Edit?"=w1189, "TeamData_and_Schedule IN"=w1185) -> ("TeamData_and_Schedule OUT"=w1186:T40, "Cancelled?"=w1187:bool)  [unwired: 3 in, 5 out]
        n743 = case shown="False" w1187 {
          tunnel: w1186 -> [w1190 _]
          frame False {
            n744 = stacked-sequence {
              tunnel: w1190 -> [w1192 _]
              frame #0 {
                n745 = Unbundle By Name(w1192) -> ("Team Info"=w1191:T41)
                n746 = stacked-sequence {
                  tunnel: [_ w1199 _] -> w1194
                  tunnel: w1191 -> [_ w1198 _]
                  frame #0 {
                    n747 = call "Team Data Control.vi"("Mode"=T24."Clear All Teams") -> ()  [unwired: 10 in, 1 out]
                  }
                  frame #1 {
                    n748 = for {
                      tunnel: w1198 -> [w1206] mode=indexing
                      tunnel: [w1205] -> w1199
                      tunnel: [w1200] -> w1197 mode=indexing
                      n749 = Unbundle By Name(w1206) -> ("Number"=w1203:u16, "Both"=w1200:string, "Name"=w1202:string, "GUID"=w1201:u16)
                      n750 = Bundle By Name(cluster=T7 {"Both"="", "Name"="", "GUID"=0, "Number"=0} ("Team Data"), "Both"=w1200, "Name"=w1202, "Number"=w1203, "GUID"=w1201) -> (w1207:T7)
                      n751 = call "Team Data Control.vi"("Team Data To Add/Change"=w1207, "Mode"=T39."Add Team With GUID") -> ("Team Array Out"=w1205:T7[])  [unwired: 9 in]
                    }
                    n752 = property on="Select a Team for Manual Score Entry" class="Ring (strict)"("Strings []"=w1197) -> ()  [unwired: 2 in, 2 out]
                  }
                  frame #2 {
                    n753 = local read "Select a Team for Manual Score Entry"() -> (w1213:u16)
                    n754 = property on="Select a Team for Manual Score Entry" class="Ring (strict)"() -> ("Strings []"=w1214:string[])  [unwired: 2 in, 2 out]
                    n755 = Index Array(array=w1214, index=w1213) -> (element=w1211:string)
                    n756 = Decimal String To Number(string=w1211) -> (number=w1212:i32)  [unwired: 2 in, 1 out]
                    n757 = call "Get_Next_Round.vi"("TeamNo"=w1212) -> ("NextRound"=w1210:u16)  [unwired: 10 in]
                    n758 = Decrement(x=w1210) -> (x-1=w1209:u16)
                    n759 = local write "ROUND"(w1209) -> ()
                  }
                }
                n760 = local read "Team Data File Path"() -> (w1193:path)
                n761 = Flatten To XML(anything=w1194) -> (xml string=w1195:string)
                n762 = call-poly <vilib>:"Write to XML File.vi"("XML Input"=w1195, "XML File Path"=w1193) -> ()  [unwired: 7 in, 3 out]
              }
              frame #1 {
                w1215 = T21."Enabled" ("Disabled")
                n763 = local write "Startup Navigation Tab Control"(enum32{"Start", "New", "Done"}."Done" ("Startup Navigation Tab Control")) -> ()
                n764 = property on="Launch Score Entry" class="Bool (strict)"("DisabledEnum"=w1215) -> ()  [unwired: 2 in, 2 out]
                n765 = property on="Go to Timekeeper Button" class="Bool (strict)"("DisabledEnum"=w1215) -> ()  [unwired: 2 in, 2 out]
                n766 = property on="Settings Button" class="Bool (strict)"("DisabledEnum"=w1215) -> ()  [unwired: 2 in, 2 out]
                n767 = property on="System Monitor Button" class="Bool (strict)"("DisabledEnum"=w1215) -> ()  [unwired: 2 in, 2 out]
                n768 = property on="View Rankings Button" class="Bool (strict)"("DisabledEnum"=w1215) -> ()  [unwired: 2 in, 2 out]
                n769 = property on="Profile Button" class="Bool (strict)"("DisabledEnum"=w1215) -> ()  [unwired: 2 in, 2 out]
                n770 = property on="Local Entry Button" class="Bool (strict)"("DisabledEnum"=w1215) -> ()  [unwired: 2 in, 2 out]
              }
            }
          }
          frame True {
          }
        }
      }
    }
    n771 = local read "stop"() -> (w1176:bool)
  }
